vi "Run.vi"(8 "error in (no error)":errorcluster, 11 "Channel in":refnum<class "Channel.lvclass">) -> (0 "error out":errorcluster, 3 "Channel out":refnum<class "Channel.lvclass">)   [LabVIEW 2018, in "Channel.lvclass"]
uses:
  Channel.lvclass
  C:/Users/observer/Desktop/Sparc4GUI/SPARC4_GUI/Device/Device.lvclass
  Channel.lvclass/Channel.ctl
  Interface/Interface.lvclass/Interface.ctl
  Device/Device.lvclass/Device.ctl
  StateMachine/State Machine.lvclass
  Interface/Interface.lvclass
  Device/Device.lvclass
panel:
  out "x = y?":T1
  out "resp ABORT":string
  out "resp STOP":string
  out "resposta do STATUS":string
  out "resp INIT":string
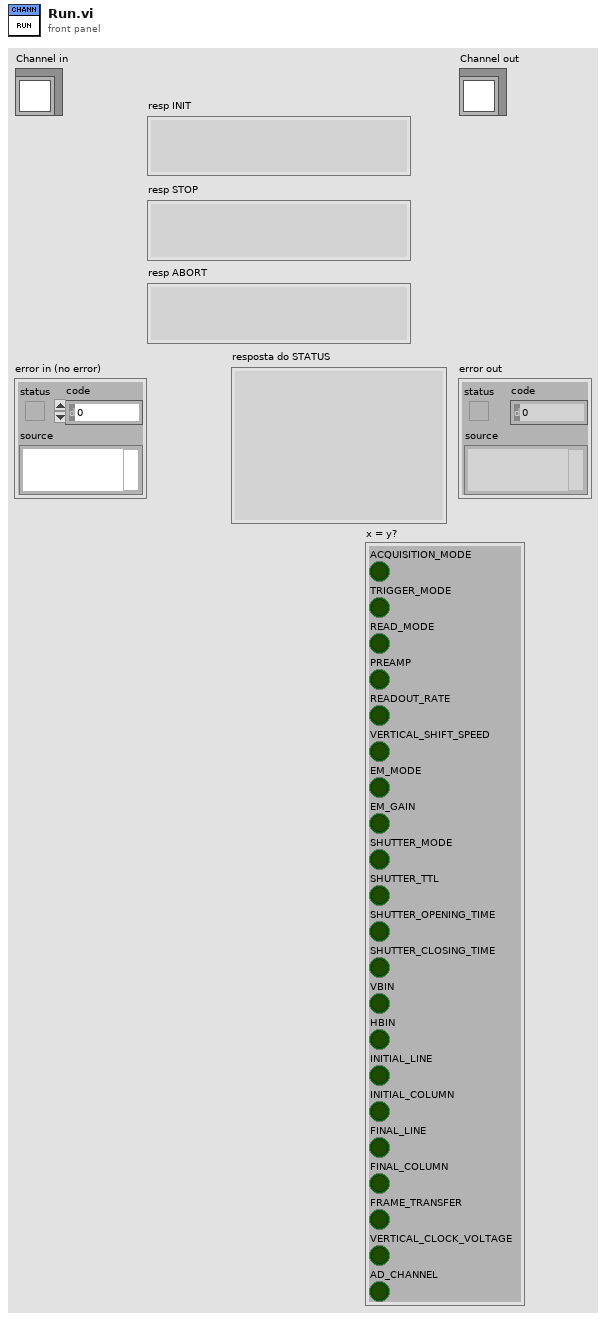
[diagram p1: front panel]
types:
  T1 = cluster{"ACQUISITION_MODE":bool, "TRIGGER_MODE":bool, "READ_MODE":bool, "PREAMP":bool, "READOUT_RATE":bool, "VERTICAL_SHIFT_SPEED":bool, "EM_MODE":bool, "EM_GAIN":bool, "SHUTTER_MODE":bool, "SHUTTER_TTL":bool, "SHUTTER_OPENING_TIME":bool, "SHUTTER_CLOSING_TIME":bool, "VBIN":bool, "HBIN":bool, "INITIAL_LINE":bool, "INITIAL_COLUMN":bool, "FINAL_LINE":bool, "FINAL_COLUMN":bool, "FRAME_TRANSFER":bool, "VERTICAL_CLOCK_VOLTAGE":bool, "AD_CHANNEL":bool}
  T2 = cluster{"ACQUISITION_MODE":u8, "TRIGGER_MODE":u8, "READ_MODE":u8, "PREAMP":u8, "READOUT_RATE":u8, "VERTICAL_SHIFT_SPEED":u8, "EM_MODE":u8, "EM_GAIN":u16, "SHUTTER_MODE":u8, "SHUTTER_TTL":u8, "SHUTTER_OPENING_TIME":u16, "SHUTTER_CLOSING_TIME":u16, "VBIN":u16, "HBIN":u16, "INITIAL_LINE":u16, "INITIAL_COLUMN":u16, "FINAL_LINE":u16, "FINAL_COLUMN":u16, "FRAME_TRANSFER":bool, "VERTICAL_CLOCK_VOLTAGE":u8, "AD_CHANNEL":u32}
  T3 = cluster{"Image Name":string, "Image Path":string, "#FRAMES":u32, "EXPTIME":dbl, "PREAMP":u8, "READOUT_RATE":u8, "VERTICAL_SHIFT_SPEED":u8, "ACQUISITION_MODE":u8, "READ_MODE":u8, "EM_MODE":u8, "EM_GAIN":u16, "SHUTTER_MODE":u8, "SHUTTER_TTL":u8, "SHUTTER_OPENNING_TIME":u16, "SHUTTER_CLOSING_TIME":u16, "VBIN":u16, "HBIN":u16, "INITIAL_LINE":u16, "INITIAL_COLUMN":u16, "FINAL_LINE":u16, "FINAL_COLUMN":u16, "Cooler ON/OFF":u16, "Set temperature":i8, "Exposições realizadas":u16, "Kinetic Serie Length":u32, "Number of Accumulations":u32, "Kinetic Cycle Time":u32, "FRAME_TRANSFER":bool, "VERTICAL_CLOCK_VOLTAGE":u8, "TRIGGER_MODE":u8, "Number of exp":u32, "AD_CHANNEL":u32}
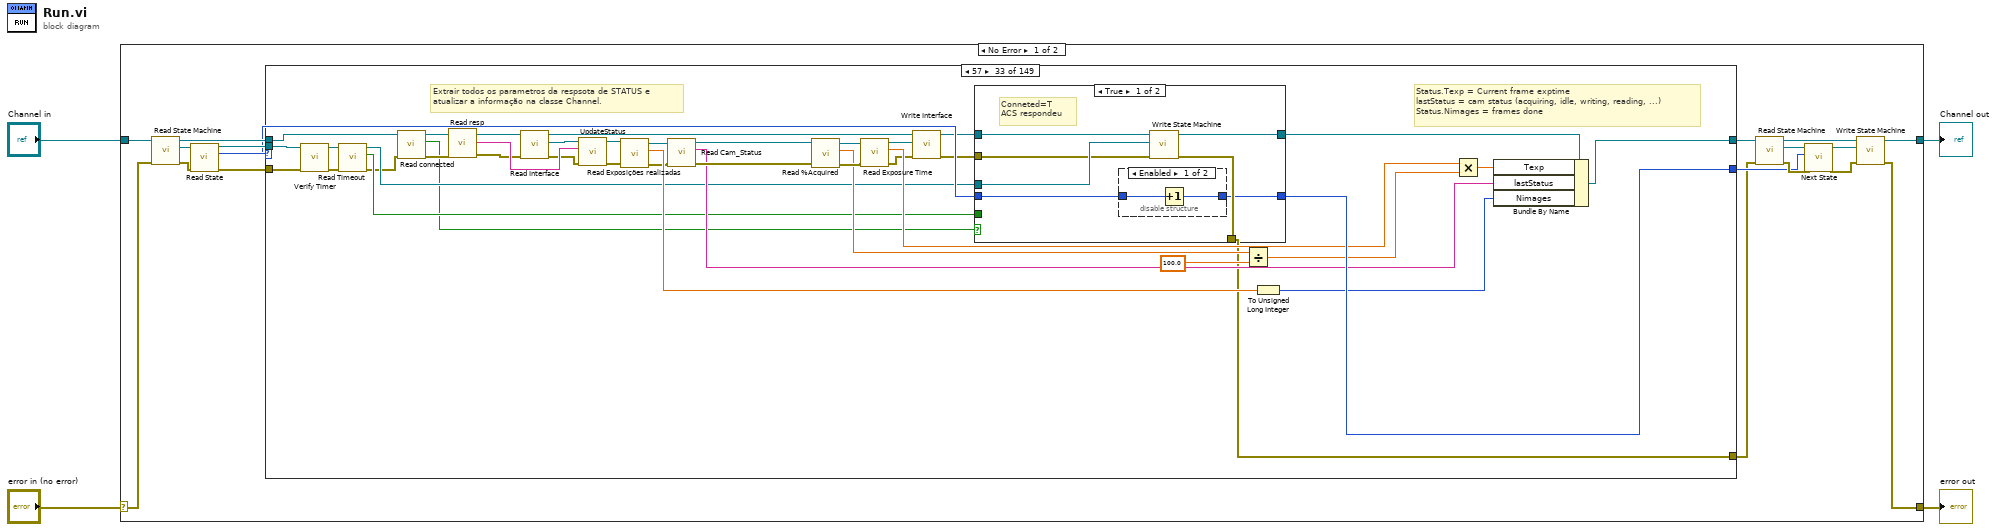
[diagram p0: block diagram]
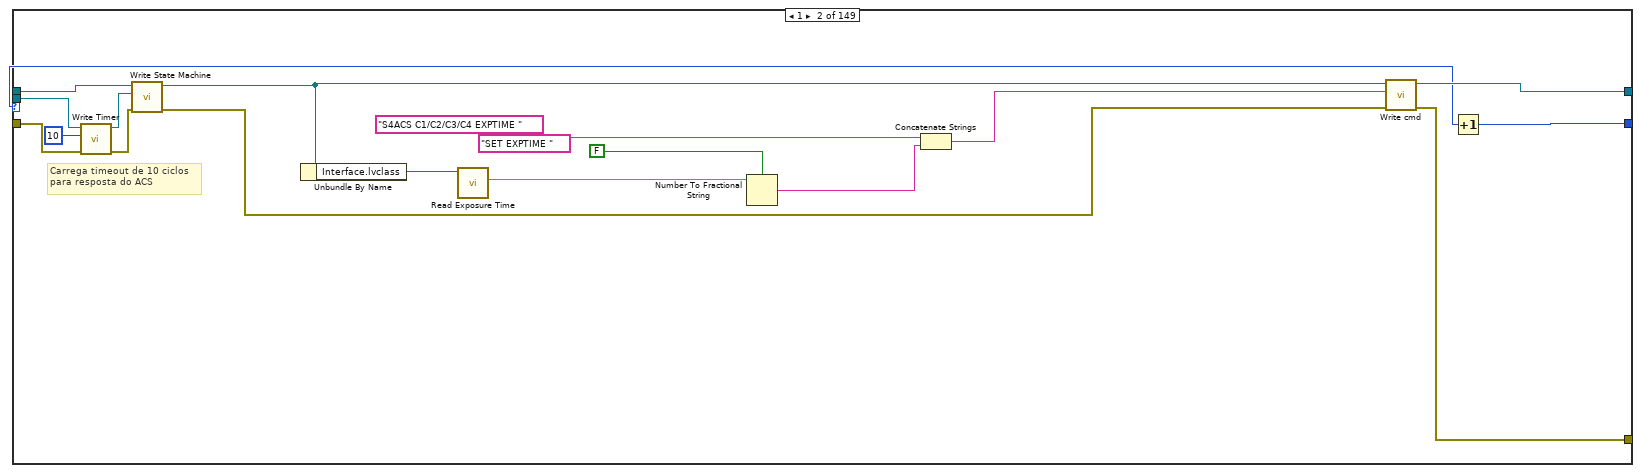
[diagram p3: hidden frame]
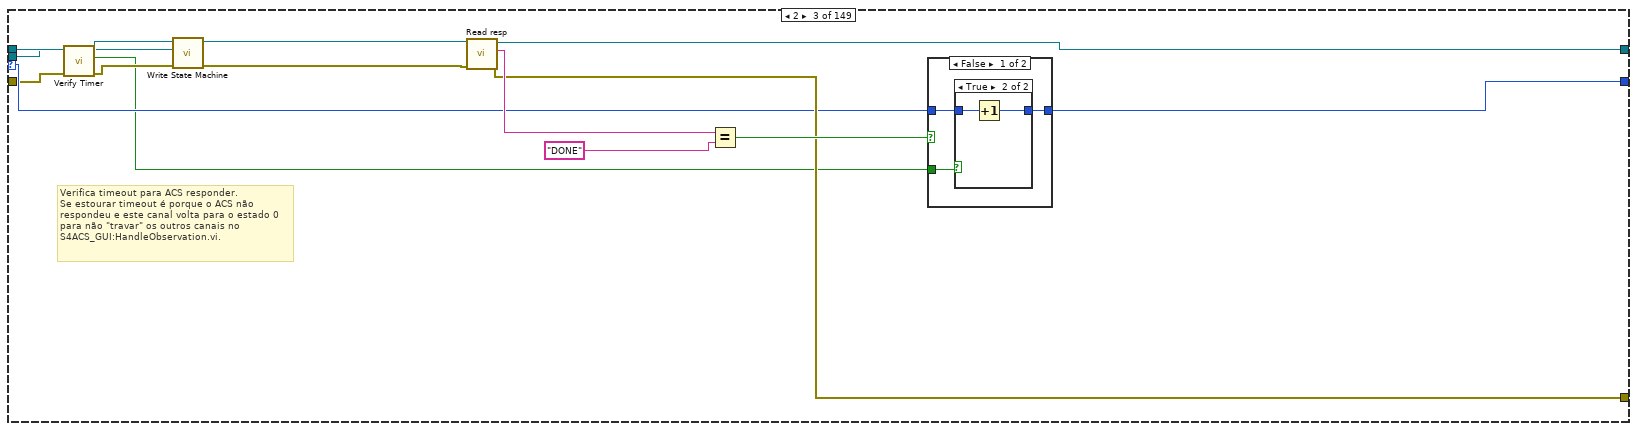
[diagram p4: hidden frame]
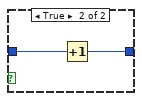
[diagram p6: hidden frame]
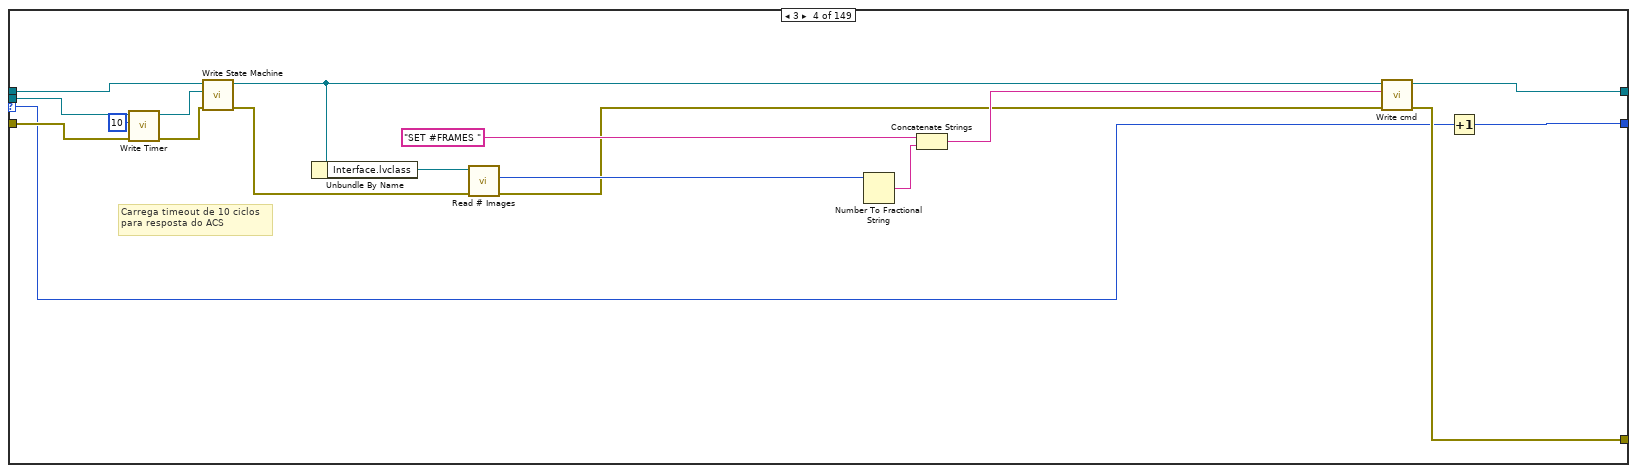
[diagram p7: hidden frame]
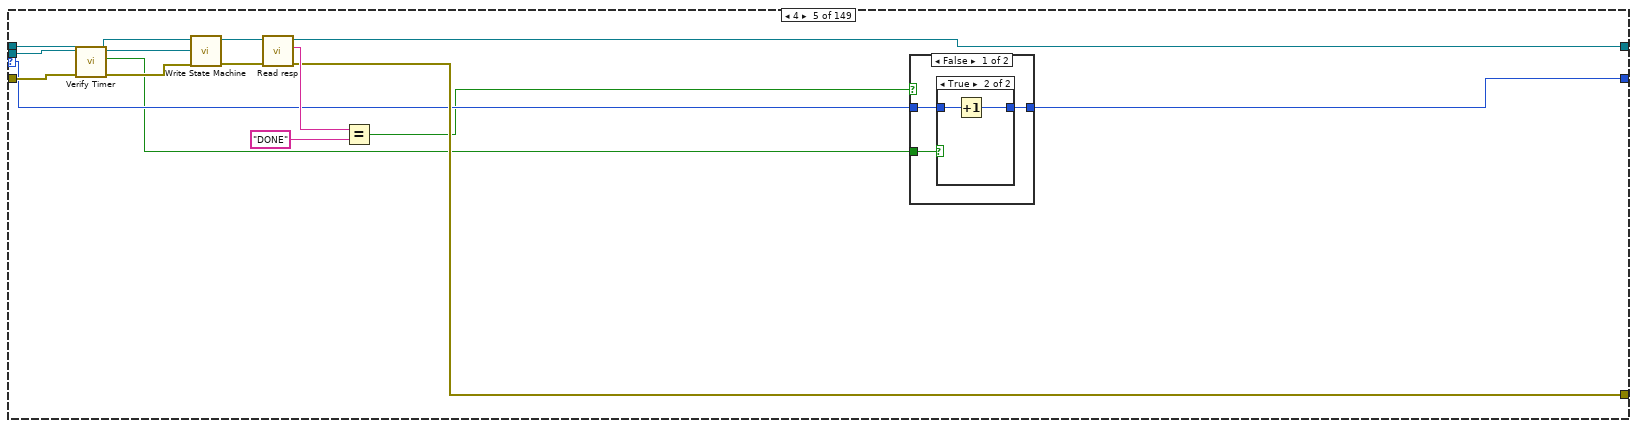
[diagram p8: hidden frame]
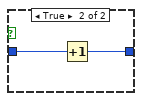
[diagram p10: hidden frame]
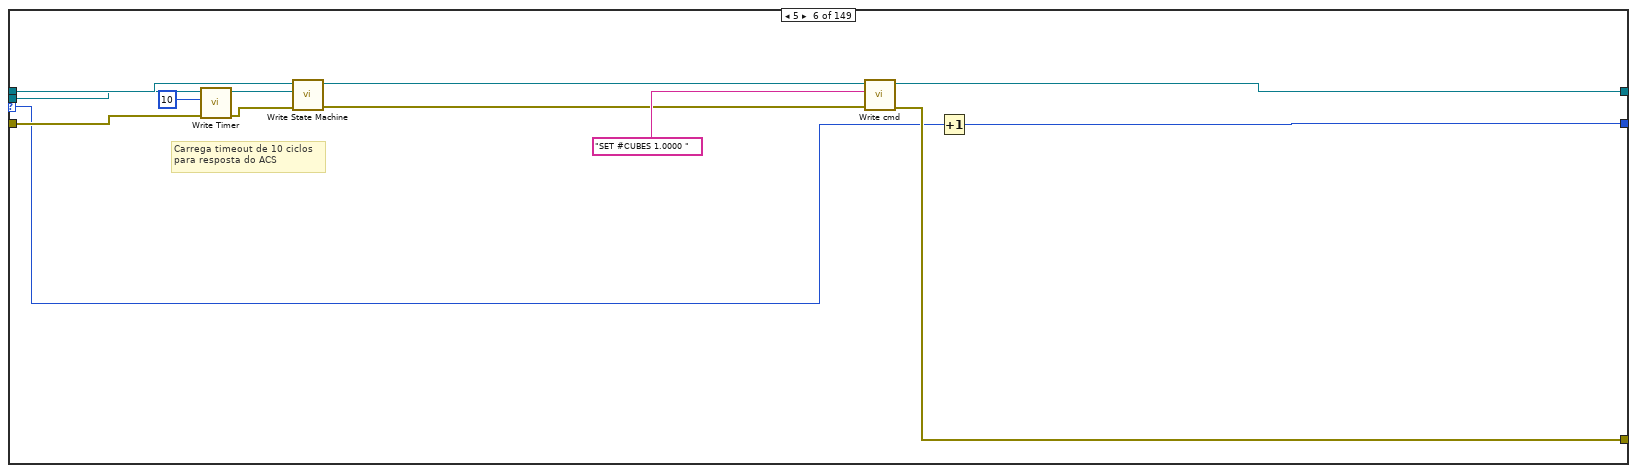
[diagram p11: hidden frame]
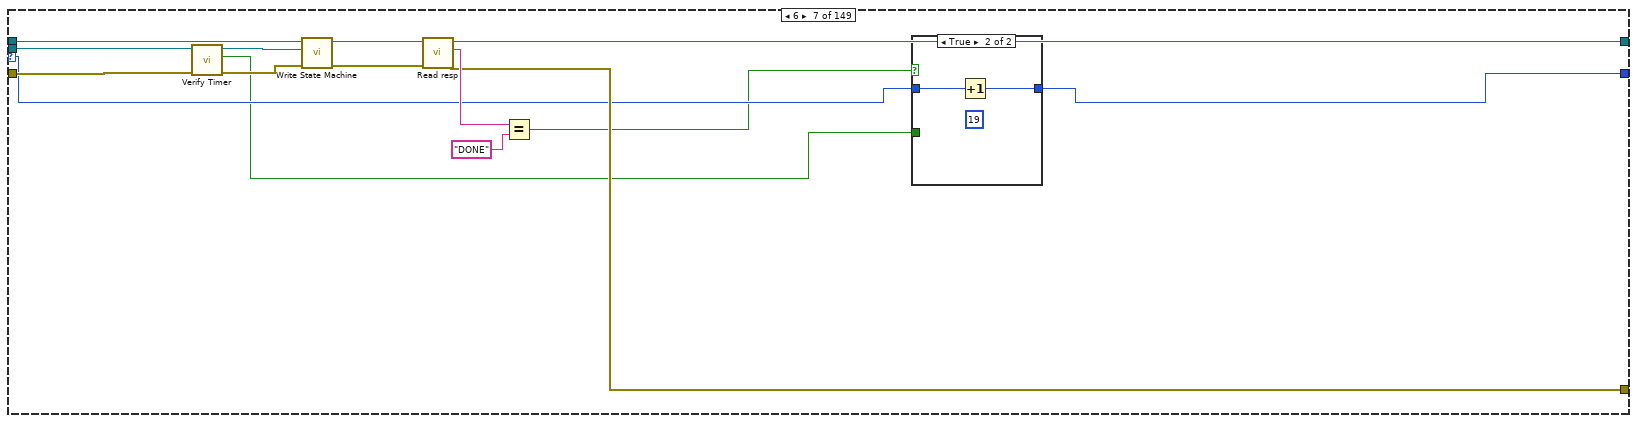
[diagram p12: hidden frame]
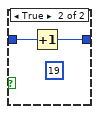
[diagram p14: hidden frame]
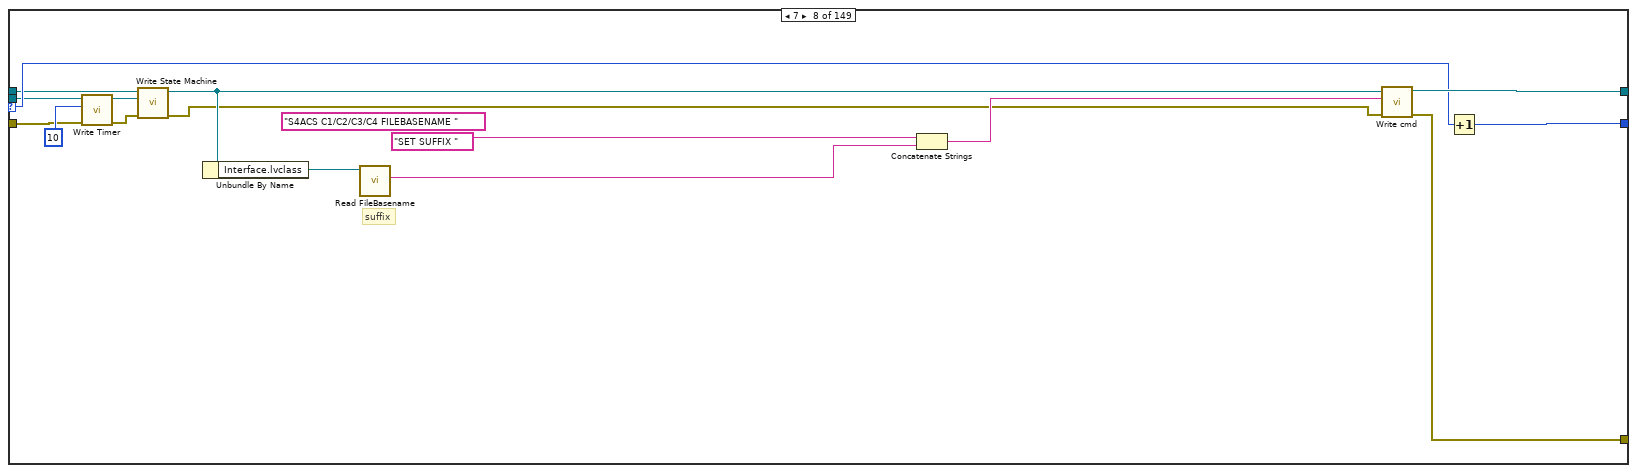
[diagram p15: hidden frame]
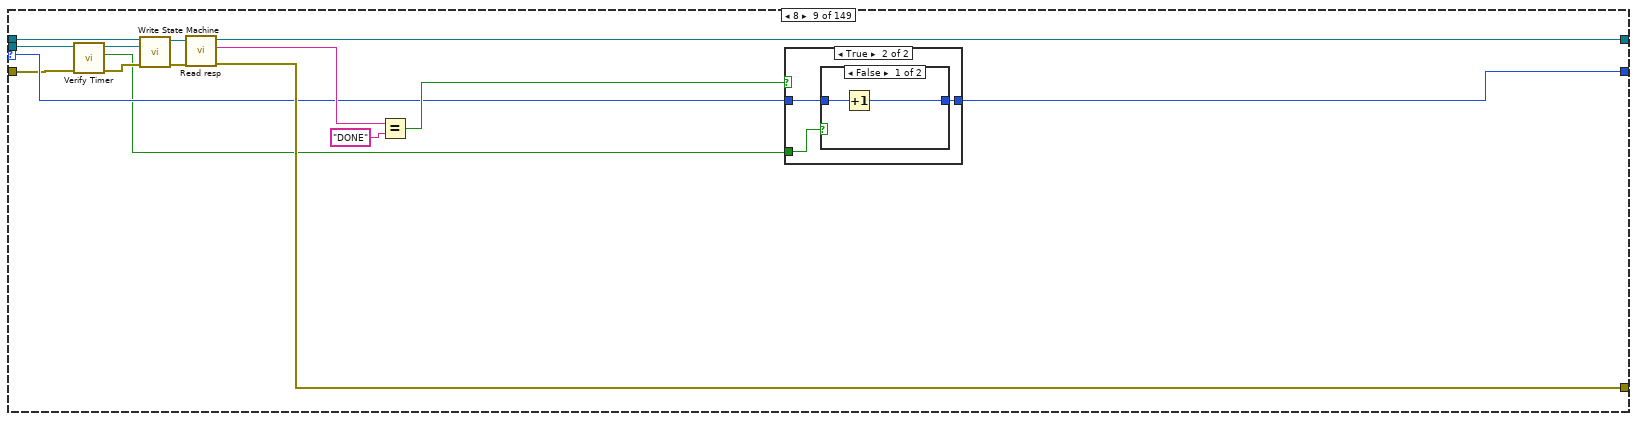
[diagram p16: hidden frame]
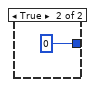
[diagram p18: hidden frame]
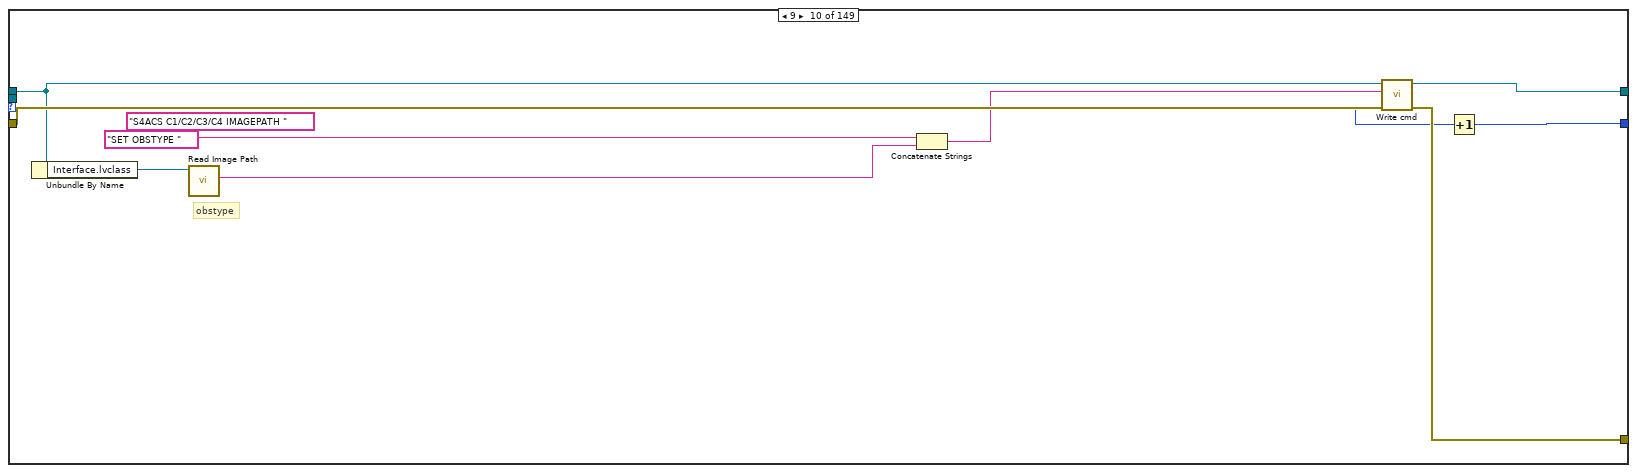
[diagram p19: hidden frame]
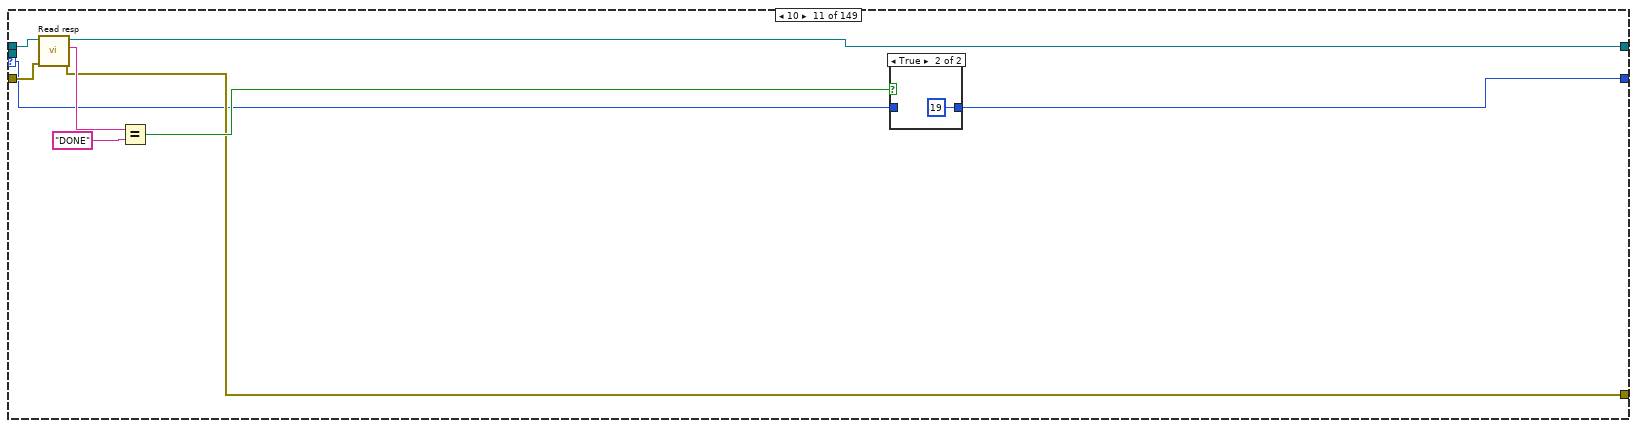
[diagram p20: hidden frame]
diagram:
  n1 = case shown="No Error" "error in (no error)" {
    selector: "error in (no error)" -> [w21 w2224]
    tunnel: [w6 w2224] -> w3
    tunnel: [w11 w2223] -> w1
    tunnel: "Channel in" -> [w22 w2223]
    frame No Error {
      n2 = call-dynamic "Read State Machine.vi"("error in (no error)"=w21, "Device in"=w22) -> ("error out"=w18:errorcluster, "State Machine.lvclass"=w20:refnum<class "State Machine.lvclass">, "Device out"=w16:refnum<class "Channel.lvclass">)  [unwired: 7 in]
      n3 = call-dynamic "Read State.vi"("error in (no error)"=w18, "State Machine in"=w20) -> ("error out"=w17:errorcluster, "State"=w19:i32, "State Machine out"=w5:refnum<class "State Machine.lvclass">)  [unwired: 7 in]
      n4 = case shown="57" w19 {
        selector: w19 -> [w25 w36 w52 w69 w88 w110 w123 w154 w168 w184 w192 w205 w213 w227 w235 w249 w257 w272 w280 w295 w311 w327 w350 w362 _ w420 w431 w445 w484 w502 w541 w598 w647 _ w729 w761 w790 w802 w816 w846 w879 w901 w925 w933 w942 w952 w961 w972 w992 w1012 w1032 w1052 w1072 w1092 w1112 w1132 _ w1152 w1160 w1173 w1186 w1202 w1210 w1223 w1237 w1249 w1257 w1270 w1283 w1295 w1303 w1316 w1329 w1341 w1349 w1362 w1375 w1387 w1395 w1408 w1421 w1433 w1441 w1454 w1467 w1479 w1487 w1500 w1513 w1525 w1533 w1546 w1559 w1575 w1583 w1596 w1609 w1621 w1629 w1642 w1655 w1667 w1675 w1688 w1701 w1713 w1721 w1734 w1747 w1759 w1767 w1780 w1793 w1805 w1813 w1826 w1839 w1851 w1859 w1872 w1885 w1897 w1905 w1918 w1931 w1943 w1951 w1964 w1977 w1989 w1997 w2010 w2023 w2035 w2043 w2056 w2069 w2085 w2093 w2106 w2119 w2131 w2141 w2154 w2167 w2181 w2189 w2202 w2215]
        tunnel: w17 -> [w24 w33 w48 w71 w90 w112 w125 w146 w166 w190 w199 w211 w220 w233 w242 w255 w264 w278 w287 w293 w303 w326 w345 w356 w407 w413 w427 w439 w449 w494 w511 w590 w617 w681 w737 w749 w784 w797 w810 w841 w876 w896 w918 w937 w946 w956 w965 w976 w987 w1007 w1027 w1047 w1067 w1087 w1107 w1127 w1145 w1158 w1167 w1177 w1189 w1208 w1217 w1227 w1240 w1255 w1264 w1274 w1286 w1301 w1310 w1320 w1332 w1347 w1356 w1366 w1378 w1393 w1402 w1412 w1424 w1439 w1448 w1458 w1470 w1485 w1494 w1504 w1516 w1531 w1540 w1550 w1562 w1581 w1590 w1600 w1612 w1627 w1636 w1646 w1658 w1673 w1682 w1692 w1704 w1719 w1728 w1738 w1750 w1765 w1774 w1784 w1796 w1811 w1820 w1830 w1842 w1857 w1866 w1876 w1888 w1903 w1912 w1922 w1934 w1949 w1958 w1968 w1980 w1995 w2004 w2014 w2026 w2041 w2050 w2060 w2072 w2091 w2100 w2110 w2122 w2137 w2148 w2158 w2170 w2187 w2196 w2206 w2218]
        tunnel: [w24 w42 w53 w83 w96 w119 w132 w158 w169 w189 w193 w210 w214 w232 w236 w254 w258 w277 w281 w293 w315 w328 w352 w364 w406 w421 w423 w447 w476 w504 w512 w586 w618 w694 w736 w762 w792 w794 w818 w826 w881 w902 w927 w934 w945 w953 w964 w973 w987 w1007 w1027 w1047 w1067 w1087 w1107 w1127 w1145 w1157 w1161 w1176 w1187 w1207 w1211 w1226 w1238 w1254 w1258 w1273 w1284 w1300 w1304 w1319 w1330 w1346 w1350 w1365 w1376 w1392 w1396 w1411 w1422 w1438 w1442 w1457 w1468 w1484 w1488 w1503 w1514 w1530 w1534 w1549 w1560 w1580 w1584 w1599 w1610 w1626 w1630 w1645 w1656 w1672 w1676 w1691 w1702 w1718 w1722 w1737 w1748 w1764 w1768 w1783 w1794 w1810 w1814 w1829 w1840 w1856 w1860 w1875 w1886 w1902 w1906 w1921 w1932 w1948 w1952 w1967 w1978 w1994 w1998 w2013 w2024 w2040 w2044 w2059 w2070 w2090 w2094 w2109 w2120 w2136 w2142 w2157 w2168 w2186 w2190 w2205 w2216] -> w7
        tunnel: w16 -> [w23 w31 w51 w72 w94 w113 w129 w148 w165 w188 w200 w209 w221 w231 w243 w253 w265 w276 w288 w292 w306 w325 w347 w359 w405 w415 w430 w441 w452 w496 w509 w592 w611 w693 w731 w753 w785 w798 w811 w842 w875 w899 w919 w938 w944 w957 w963 w977 w985 w1005 w1025 w1045 w1065 w1085 w1105 w1125 w1147 w1156 w1168 w1175 w1190 w1206 w1218 w1225 w1241 w1253 w1265 w1272 w1287 w1299 w1311 w1318 w1333 w1345 w1357 w1364 w1379 w1391 w1403 w1410 w1425 w1437 w1449 w1456 w1471 w1483 w1495 w1502 w1517 w1529 w1541 w1548 w1563 w1579 w1591 w1598 w1613 w1625 w1637 w1644 w1659 w1671 w1683 w1690 w1705 w1717 w1729 w1736 w1751 w1763 w1775 w1782 w1797 w1809 w1821 w1828 w1843 w1855 w1867 w1874 w1889 w1901 w1913 w1920 w1935 w1947 w1959 w1966 w1981 w1993 w2005 w2012 w2027 w2039 w2051 w2058 w2073 w2089 w2101 w2108 w2123 w2135 w2149 w2156 w2171 w2185 w2197 w2204 w2219]
        tunnel: [w23 w43 w54 w84 w97 w120 w133 w159 w170 w191 w194 w212 w215 w234 w237 w256 w259 w279 w282 w292 w316 w329 w353 w367 w397 w422 w424 w448 w483 w505 w540 w585 w646 w695 w738 w763 w793 w795 w819 w837 w882 w903 w928 w935 w947 w954 w966 w969 w989 w1009 w1029 w1049 w1069 w1089 w1109 w1129 w1147 w1159 w1162 w1178 w1185 w1209 w1212 w1228 w1236 w1256 w1259 w1275 w1282 w1302 w1305 w1321 w1328 w1348 w1351 w1367 w1374 w1394 w1397 w1413 w1420 w1440 w1443 w1459 w1466 w1486 w1489 w1505 w1512 w1532 w1535 w1551 w1558 w1582 w1585 w1601 w1608 w1628 w1631 w1647 w1654 w1674 w1677 w1693 w1700 w1720 w1723 w1739 w1746 w1766 w1769 w1785 w1792 w1812 w1815 w1831 w1838 w1858 w1861 w1877 w1884 w1904 w1907 w1923 w1930 w1950 w1953 w1969 w1976 w1996 w1999 w2015 w2022 w2042 w2045 w2061 w2068 w2092 w2095 w2111 w2118 w2138 w2143 w2159 w2166 w2188 w2191 w2207 w2214] -> w14
        tunnel: [w25 w37 w55 w78 w85 w118 w124 w155 w171 w185 w195 w206 w216 w228 w238 w250 w260 w273 w283 w296 w312 w330 w351 w363 w399 w410 w432 w446 w485 w503 w542 w599 w648 0 ("State") w728 w764 w791 w803 w817 w847 w880 w904 w926 w936 w943 w955 w962 w974 w984 w1004 w1024 w1044 w1064 w1084 w1104 w1124 u8 0 ("State") w1153 w1163 w1174 w1188 w1203 w1213 w1224 w1239 w1250 w1260 w1271 w1285 w1296 w1306 w1317 w1331 w1342 w1352 w1363 w1377 w1388 w1398 w1409 w1423 w1434 w1444 w1455 w1469 w1480 w1490 w1501 w1515 w1526 w1536 w1547 w1561 w1576 w1586 w1597 w1611 w1622 w1632 w1643 w1657 w1668 w1678 w1689 w1703 w1714 w1724 w1735 w1749 w1760 w1770 w1781 w1795 w1806 w1816 w1827 w1841 w1852 w1862 w1873 w1887 w1898 w1908 w1919 w1933 w1944 w1954 w1965 w1979 w1990 w2000 w2011 w2025 w2036 w2046 w2057 w2071 w2086 w2096 w2107 w2121 w2132 w2144 w2155 w2169 w2182 w2192 w2203 w2217] -> w8
        tunnel: w5 -> [_ w32 w50 w73 w95 w111 w126 w150 w167 _ _ _ _ _ _ _ _ _ _ _ w305 w323 w346 w360 _ w416 w429 w440 w454 w498 w510 w594 w616 w682 w733 w754 w787 w799 w813 w843 w877 w900 w920 _ _ _ _ _ _ _ _ _ _ _ _ _ _ _ _ _ _ _ _ _ _ _ _ _ _ _ _ _ _ _ _ _ _ _ _ _ _ _ _ _ _ _ _ _ _ _ _ _ _ _ _ _ _ _ _ _ _ _ _ _ _ _ _ _ _ _ _ _ _ _ _ _ _ _ _ _ _ _ _ _ _ _ _ _ _ _ _ _ _ _ _ _ _ _ _ _ _ _ _ _ _ _ _ _ _]
        frame 0, Default {
        }
        frame 1 {
          (unwired) "S4ACS C1/C2/C3/C4 EXPTIME " ("cmd")
          # "Carrega timeout de 10 ciclos\npara resposta do ACS"
          n5 = call-dynamic "Write Timer.vi"("error in (no error)"=w33, "Timer"=u32 10, "State Machine in"=w32) -> ("error out"=w27:errorcluster, "State Machine out"=w30:refnum<class "State Machine.lvclass">)  [unwired: 7 in]
          n6 = call-dynamic "Write State Machine.vi"("error in (no error)"=w27, "State Machine.lvclass"=w30, "Device in"=w31) -> ("error out"=w26:errorcluster, "Device out"=w29:refnum<class "Channel.lvclass">)  [unwired: 7 in]
          n7 = Unbundle By Name(w29) -> ("Interface.lvclass"=w41:refnum<class "Interface.lvclass">)
          n8 = call "Read Exposure Time.vi"("Interface in"=w41) -> ("Exposure Time"=w40:dbl)  [unwired: 8 in, 2 out]
          n9 = Number To Fractional String(use system decimal point (T)=FALSE, number=w40) -> (F-format string=w39:string)  [unwired: 2 in]
          n10 = Concatenate Strings("SET EXPTIME " ("cmd"), w39) -> (w38:string)
          n11 = call-dynamic "Write cmd.vi"("error in (no error)"=w26, "cmd"=w38, "Device in"=w29) -> ("error out"=w42:errorcluster, "Device out"=w43:refnum<class "Channel.lvclass">)  [unwired: 7 in]
          n12 = Increment(x=w36) -> (x+1=w37:i32)
        }
        frame 2 {
          # "Verifica timeout para ACS responder.\nSe estourar timeout é porque o ACS não \nrespondeu e este canal volta para o estado 0\npara não \"travar\" os outros canais no \nS4ACS_GUI:HandleObservation.vi."
          n13 = call "Verify Timer.vi"("error in (no error)"=w48, "State Machine in"=w50) -> ("error out"=w47:errorcluster, "timeout"=w44:bool, "State Machine out"=w49:refnum<class "State Machine.lvclass">)  [unwired: 7 in]
          n14 = call-dynamic "Write State Machine.vi"("error in (no error)"=w47, "State Machine.lvclass"=w49, "Device in"=w51) -> ("error out"=w46:errorcluster, "Device out"=w45:refnum<class "Channel.lvclass">)  [unwired: 7 in]
          n15 = call-dynamic "Read resp.vi"("error in (no error)"=w46, "Device in"=w45) -> ("error out"=w53:errorcluster, "resp"=w58:string, "Device out"=w54:refnum<class "Channel.lvclass">)  [unwired: 7 in]
          n16 = Equal?(x=w58, y="DONE") -> (x = y?=w56:bool)
          n17 = case shown="False" w56 {
            tunnel: [w60 w65] -> w55
            tunnel: w52 -> [w61 w66]
            tunnel: w44 -> [w59 _]
            frame False {
              n18 = case shown="True" w59 {
                tunnel: [w62 w63] -> w60
                tunnel: w61 -> [w62 w64]
                frame False {
                }
                frame True {
                  n19 = Increment(x=w64) -> (x+1=w63:i32)
                }
              }
            }
            frame True {
              n20 = Increment(x=w66) -> (x+1=w65:i32)
            }
          }
        }
        frame 3 {
          # "Carrega timeout de 10 ciclos\npara resposta do ACS"
          n21 = call-dynamic "Write Timer.vi"("error in (no error)"=w71, "Timer"=u32 10, "State Machine in"=w73) -> ("error out"=w74:errorcluster, "State Machine out"=w76:refnum<class "State Machine.lvclass">)  [unwired: 7 in]
          n22 = call-dynamic "Write State Machine.vi"("error in (no error)"=w74, "State Machine.lvclass"=w76, "Device in"=w72) -> ("error out"=w68:errorcluster, "Device out"=w70:refnum<class "Channel.lvclass">)  [unwired: 7 in]
          n23 = Unbundle By Name(w70) -> ("Interface.lvclass"=w82:refnum<class "Interface.lvclass">)
          n24 = call-dynamic "Read # Images.vi"("error in (no error)"=w68, "Interface in"=w82) -> ("error out"=w67:errorcluster, "# Images"=w81:u32)  [unwired: 7 in, 1 out]
          n25 = Number To Fractional String(number=w81) -> (F-format string=w80:string)  [unwired: 3 in]
          n26 = Concatenate Strings("SET #FRAMES " ("cmd"), w80) -> (w79:string)
          n27 = call-dynamic "Write cmd.vi"("error in (no error)"=w67, "cmd"=w79, "Device in"=w70) -> ("error out"=w83:errorcluster, "Device out"=w84:refnum<class "Channel.lvclass">)  [unwired: 7 in]
          n28 = Increment(x=w69) -> (x+1=w78:i32)
        }
        frame 4 {
          n29 = call "Verify Timer.vi"("error in (no error)"=w90, "State Machine in"=w95) -> ("error out"=w89:errorcluster, "timeout"=w86:bool, "State Machine out"=w91:refnum<class "State Machine.lvclass">)  [unwired: 7 in]
          n30 = call-dynamic "Write State Machine.vi"("error in (no error)"=w89, "State Machine.lvclass"=w91, "Device in"=w94) -> ("error out"=w92:errorcluster, "Device out"=w93:refnum<class "Channel.lvclass">)  [unwired: 7 in]
          n31 = call-dynamic "Read resp.vi"("error in (no error)"=w92, "Device in"=w93) -> ("error out"=w96:errorcluster, "resp"=w99:string, "Device out"=w97:refnum<class "Channel.lvclass">)  [unwired: 7 in]
          n32 = Equal?(x=w99, y="DONE") -> (x = y?=w87:bool)
          n33 = case shown="False" w87 {
            tunnel: [w101 w106] -> w85
            tunnel: w88 -> [w102 w107]
            tunnel: w86 -> [w100 _]
            frame False {
              n34 = case shown="True" w100 {
                tunnel: [w103 w104] -> w101
                tunnel: w102 -> [w103 w105]
                frame False {
                }
                frame True {
                  n35 = Increment(x=w105) -> (x+1=w104:i32)
                }
              }
            }
            frame True {
              n36 = Increment(x=w107) -> (x+1=w106:i32)
            }
          }
        }
        frame 5 {
          # "Carrega timeout de 10 ciclos\npara resposta do ACS"
          n37 = call-dynamic "Write Timer.vi"("error in (no error)"=w112, "Timer"=u32 10, "State Machine in"=w111) -> ("error out"=w114:errorcluster, "State Machine out"=w116:refnum<class "State Machine.lvclass">)  [unwired: 7 in]
          n38 = call-dynamic "Write State Machine.vi"("error in (no error)"=w114, "State Machine.lvclass"=w116, "Device in"=w113) -> ("error out"=w109:errorcluster, "Device out"=w108:refnum<class "Channel.lvclass">)  [unwired: 7 in]
          n39 = call-dynamic "Write cmd.vi"("error in (no error)"=w109, "cmd"="SET #CUBES 1.0000 ", "Device in"=w108) -> ("error out"=w119:errorcluster, "Device out"=w120:refnum<class "Channel.lvclass">)  [unwired: 7 in]
          n40 = Increment(x=w110) -> (x+1=w118:i32)
        }
        frame 6 {
          n41 = call "Verify Timer.vi"("error in (no error)"=w125, "State Machine in"=w126) -> ("error out"=w130:errorcluster, "timeout"=w121:bool, "State Machine out"=w131:refnum<class "State Machine.lvclass">)  [unwired: 7 in]
          n42 = call-dynamic "Write State Machine.vi"("error in (no error)"=w130, "State Machine.lvclass"=w131, "Device in"=w129) -> ("error out"=w127:errorcluster, "Device out"=w128:refnum<class "Channel.lvclass">)  [unwired: 7 in]
          n43 = call-dynamic "Read resp.vi"("error in (no error)"=w127, "Device in"=w128) -> ("error out"=w132:errorcluster, "resp"=w135:string, "Device out"=w133:refnum<class "Channel.lvclass">)  [unwired: 7 in]
          n44 = Equal?(x=w135, y="DONE") -> (x = y?=w122:bool)
          n45 = case shown="True" w122 {
            tunnel: [w137 w142] -> w124
            tunnel: w123 -> [w138 w143]
            tunnel: w121 -> [w136 _]
            frame False {
              n46 = case shown="False" w136 {
                tunnel: [w139 w140] -> w137
                tunnel: w138 -> [w139 w141]
                frame False {
                }
                frame True {
                  (unwired) 19 ("State")
                  n47 = Increment(x=w141) -> (x+1=w140:i32)
                }
              }
            }
            frame True {
              (unwired) 19
              n48 = Increment(x=w143) -> (x+1=w142:i32)
            }
          }
        }
        frame 7 {
          (unwired) "S4ACS C1/C2/C3/C4 FILEBASENAME " ("cmd")
          # "suffix"
          n49 = call-dynamic "Write Timer.vi"("error in (no error)"=w146, "Timer"=u32 10, "State Machine in"=w150) -> ("error out"=w151:errorcluster, "State Machine out"=w144:refnum<class "State Machine.lvclass">)  [unwired: 7 in]
          n50 = call-dynamic "Write State Machine.vi"("error in (no error)"=w151, "State Machine.lvclass"=w144, "Device in"=w148) -> ("error out"=w145:errorcluster, "Device out"=w147:refnum<class "Channel.lvclass">)  [unwired: 7 in]
          n51 = Unbundle By Name(w147) -> ("Interface.lvclass"=w157:refnum<class "Interface.lvclass">)
          n52 = call-dynamic "Read FileBasename.vi"("Interface in"=w157) -> ("FileBasename"=w152:string)  [unwired: 8 in, 2 out]
          n53 = Concatenate Strings("SET SUFFIX " ("cmd"), w152) -> (w156:string)
          n54 = call-dynamic "Write cmd.vi"("error in (no error)"=w145, "cmd"=w156, "Device in"=w147) -> ("error out"=w158:errorcluster, "Device out"=w159:refnum<class "Channel.lvclass">)  [unwired: 7 in]
          n55 = Increment(x=w154) -> (x+1=w155:i32)
        }
        frame 8 {
          n56 = call "Verify Timer.vi"("error in (no error)"=w166, "State Machine in"=w167) -> ("error out"=w163:errorcluster, "timeout"=w160:bool, "State Machine out"=w164:refnum<class "State Machine.lvclass">)  [unwired: 7 in]
          n57 = call-dynamic "Write State Machine.vi"("error in (no error)"=w163, "State Machine.lvclass"=w164, "Device in"=w165) -> ("error out"=w162:errorcluster, "Device out"=w161:refnum<class "Channel.lvclass">)  [unwired: 7 in]
          n58 = call-dynamic "Read resp.vi"("error in (no error)"=w162, "Device in"=w161) -> ("error out"=w169:errorcluster, "resp"=w174:string, "Device out"=w170:refnum<class "Channel.lvclass">)  [unwired: 7 in]
          n59 = Equal?(x=w174, y="DONE") -> (x = y?=w172:bool)
          n60 = case shown="True" w172 {
            tunnel: [w175 w177] -> w171
            tunnel: w168 -> [w175 w178]
            tunnel: w160 -> [_ w176]
            frame False {
            }
            frame True {
              n61 = case shown="False" w176 {
                tunnel: w178 -> [w180 _]
                tunnel: [w179 0] -> w177
                frame False {
                  n62 = Increment(x=w180) -> (x+1=w179:i32)
                }
                frame True {
                }
              }
            }
          }
        }
        frame 9 {
          (unwired) "S4ACS C1/C2/C3/C4 IMAGEPATH " ("cmd")
          # "obstype"
          n63 = Unbundle By Name(w188) -> ("Interface.lvclass"=w187:refnum<class "Interface.lvclass">)
          n64 = call-dynamic "Read Image Path.vi"("Interface in"=w187) -> ("Image Path"=w182:string)  [unwired: 8 in, 2 out]
          n65 = Concatenate Strings("SET OBSTYPE " ("cmd"), w182) -> (w186:string)
          n66 = call-dynamic "Write cmd.vi"("error in (no error)"=w190, "cmd"=w186, "Device in"=w188) -> ("error out"=w189:errorcluster, "Device out"=w191:refnum<class "Channel.lvclass">)  [unwired: 7 in]
          n67 = Increment(x=w184) -> (x+1=w185:i32)
        }
        frame 10 {
          n68 = call-dynamic "Read resp.vi"("error in (no error)"=w199, "Device in"=w200) -> ("error out"=w193:errorcluster, "resp"=w198:string, "Device out"=w194:refnum<class "Channel.lvclass">)  [unwired: 7 in]
          n69 = Equal?(x=w198, y="DONE") -> (x = y?=w196:bool)
          n70 = case shown="True" w196 {
            tunnel: [w201 19 ("State")] -> w195
            tunnel: w192 -> [w201 _]
            frame False {
            }
            frame True {
            }
          }
        }
        frame 11 {
          (unwired) "S4ACS C1/C2/C3/C4 OBSTITLE " ("cmd")
          n71 = Unbundle By Name(w209) -> ("Interface.lvclass"=w208:refnum<class "Interface.lvclass">)
          n72 = call-dynamic "Read ObsTitle.vi"("Interface in"=w208) -> ("ObsTitle"=w203:string)  [unwired: 8 in, 2 out]
          n73 = Concatenate Strings("SET OBSERVATION_TITLE " ("cmd"), w203) -> (w207:string)
          n74 = call-dynamic "Write cmd.vi"("error in (no error)"=w211, "cmd"=w207, "Device in"=w209) -> ("error out"=w210:errorcluster, "Device out"=w212:refnum<class "Channel.lvclass">)  [unwired: 7 in]
          n75 = Increment(x=w205) -> (x+1=w206:i32)
        }
        frame 12 {
          n76 = call-dynamic "Read resp.vi"("error in (no error)"=w220, "Device in"=w221) -> ("error out"=w214:errorcluster, "resp"=w219:string, "Device out"=w215:refnum<class "Channel.lvclass">)  [unwired: 7 in]
          n77 = Equal?(x=w219, y="DONE") -> (x = y?=w217:bool)
          n78 = case shown="True" w217 {
            tunnel: [w222 w223] -> w216
            tunnel: w213 -> [w222 w224]
            frame False {
            }
            frame True {
              n79 = Increment(x=w224) -> (x+1=w223:i32)
            }
          }
        }
        frame 13 {
          (unwired) "S4ACS C1/C2/C3/C4 COMMENTS " ("cmd")
          n80 = Unbundle By Name(w231) -> ("Interface.lvclass"=w230:refnum<class "Interface.lvclass">)
          n81 = call-dynamic "Read Comments.vi"("Interface in"=w230) -> ("Comments"=w225:string)  [unwired: 8 in, 2 out]
          n82 = Concatenate Strings("SET COMMENT " ("cmd"), w225) -> (w229:string)
          n83 = call-dynamic "Write cmd.vi"("error in (no error)"=w233, "cmd"=w229, "Device in"=w231) -> ("error out"=w232:errorcluster, "Device out"=w234:refnum<class "Channel.lvclass">)  [unwired: 7 in]
          n84 = Increment(x=w227) -> (x+1=w228:i32)
        }
        frame 14 {
          n85 = call-dynamic "Read resp.vi"("error in (no error)"=w242, "Device in"=w243) -> ("error out"=w236:errorcluster, "resp"=w241:string, "Device out"=w237:refnum<class "Channel.lvclass">)  [unwired: 7 in]
          n86 = Equal?(x=w241, y="DONE") -> (x = y?=w239:bool)
          n87 = case shown="True" w239 {
            tunnel: [w244 w245] -> w238
            tunnel: w235 -> [w244 w246]
            frame False {
            }
            frame True {
              n88 = Increment(x=w246) -> (x+1=w245:i32)
            }
          }
        }
        frame 15 {
          (unwired) "S4ACS C1/C2/C3/C4 DS9 " ("cmd")
          n89 = Unbundle By Name(w253) -> ("Interface.lvclass"=w252:refnum<class "Interface.lvclass">)
          n90 = call-dynamic "Read DS9.vi"("Interface in"=w252) -> ("DS9"=w247:string)  [unwired: 8 in, 2 out]
          n91 = Concatenate Strings("SET DS9 " ("cmd"), w247) -> (w251:string)
          n92 = call-dynamic "Write cmd.vi"("error in (no error)"=w255, "cmd"=w251, "Device in"=w253) -> ("error out"=w254:errorcluster, "Device out"=w256:refnum<class "Channel.lvclass">)  [unwired: 7 in]
          n93 = Increment(x=w249) -> (x+1=w250:i32)
        }
        frame 16 {
          n94 = call-dynamic "Read resp.vi"("error in (no error)"=w264, "Device in"=w265) -> ("error out"=w258:errorcluster, "resp"=w263:string, "Device out"=w259:refnum<class "Channel.lvclass">)  [unwired: 7 in]
          n95 = Equal?(x=w263, y="DONE") -> (x = y?=w261:bool)
          n96 = case shown="True" w261 {
            tunnel: [w266 w267] -> w260
            tunnel: w257 -> [w266 w268]
            frame False {
            }
            frame True {
              n97 = Increment(x=w268) -> (x+1=w267:i32)
            }
          }
        }
        frame 17 {
          (unwired) "S4ACS C1/C2/C3/C4 DS9 " ("cmd")
          n98 = Unbundle By Name(w276) -> ("Interface.lvclass"=w275:refnum<class "Interface.lvclass">)
          n99 = call "Read Kinetic Series Length.vi"("Interface in"=w275) -> ("Kinetic Series Length"=w270:u32)  [unwired: 8 in, 2 out]
          n100 = Number To Decimal String(number=w270) -> (decimal integer string=w269:string)  [unwired: 1 in]
          n101 = Concatenate Strings("SET KSERLEN " ("cmd"), w269) -> (w274:string)
          n102 = call-dynamic "Write cmd.vi"("error in (no error)"=w278, "cmd"=w274, "Device in"=w276) -> ("error out"=w277:errorcluster, "Device out"=w279:refnum<class "Channel.lvclass">)  [unwired: 7 in]
          n103 = Increment(x=w272) -> (x+1=w273:i32)
        }
        frame 18 {
          n104 = call-dynamic "Read resp.vi"("error in (no error)"=w287, "Device in"=w288) -> ("error out"=w281:errorcluster, "resp"=w286:string, "Device out"=w282:refnum<class "Channel.lvclass">)  [unwired: 7 in]
          n105 = Equal?(x=w286, y="DONE") -> (x = y?=w284:bool)
          n106 = case shown="True" w284 {
            tunnel: [w289 w290] -> w283
            tunnel: w280 -> [w289 w291]
            frame False {
            }
            frame True {
              n107 = Increment(x=w291) -> (x+1=w290:i32)
            }
          }
        }
        frame 19 {
          n108 = Unbundle By Name(w292) -> ("expose"=w294:bool)
          n109 = case shown="False" w294 {
            tunnel: [u8 0 ("State") u8 50 ("State")] -> w296
            tunnel: w295 -> [_ _]
            frame False {
            }
            frame True {
            }
          }
        }
        frame 30 {
          n110 = call-dynamic "Write Timer.vi"("error in (no error)"=w303, "Timer"=u32 50, "State Machine in"=w305) -> ("error out"=w302:errorcluster, "State Machine out"=w304:refnum<class "State Machine.lvclass">)  [unwired: 7 in]
          n111 = call-dynamic "Write State Machine.vi"("error in (no error)"=w302, "State Machine.lvclass"=w304, "Device in"=w306) -> ("error out"=w300:errorcluster, "Device out"=w301:refnum<class "Channel.lvclass">)  [unwired: 7 in]
          n112 = Unbundle By Name(w301) -> ("Interface.lvclass"=w314:refnum<class "Interface.lvclass">)
          n113 = call-dynamic "Read Cooler ON_OFF.vi"("error in (no error)"=w300, "Interface in"=w314) -> ("error out"=w299:errorcluster, "Cooler ON/OFF"=w309:i16)  [unwired: 7 in, 1 out]
          n114 = case shown="1, Default" w309 {
            tunnel: ["1" "0"] -> w308
            frame 0 {
              (unwired) "ON"
              # "Se COOLER desligado, manda ligar."
            }
            frame 1, Default {
              (unwired) "OFF"
              # "Se COOLER ligado, manda desligar."
            }
          }
          n115 = Concatenate Strings("SET COOLER_POWER_STATUS " ("cmd"), w308) -> (w313:string)
          n116 = call-dynamic "Write cmd.vi"("error in (no error)"=w299, "cmd"=w313, "Device in"=w301) -> ("error out"=w315:errorcluster, "Device out"=w316:refnum<class "Channel.lvclass">)  [unwired: 7 in]
          n117 = Increment(x=w311) -> (x+1=w312:i32)
        }
        frame 31 {
          n118 = call "Verify Timer.vi"("error in (no error)"=w326, "State Machine in"=w323) -> ("error out"=w321:errorcluster, "timeout"=w319:bool, "State Machine out"=w322:refnum<class "State Machine.lvclass">)  [unwired: 7 in]
          n119 = call-dynamic "Write State Machine.vi"("error in (no error)"=w321, "State Machine.lvclass"=w322, "Device in"=w325) -> ("error out"=w320:errorcluster, "Device out"=w324:refnum<class "Channel.lvclass">)  [unwired: 7 in]
          n120 = call-dynamic "Read resp.vi"("error in (no error)"=w320, "Device in"=w324) -> ("error out"=w328:errorcluster, "resp"=w333:string, "Device out"=w329:refnum<class "Channel.lvclass">)  [unwired: 7 in]
          n121 = Equal?(x=w333, y="DONE") -> (x = y?=w331:bool)
          n122 = case shown="False" w319 {
            tunnel: w331 -> [w336 _]
            tunnel: [w335 0 ("State")] -> w330
            tunnel: w327 -> [w334 _]
            frame False {
              n123 = case shown="True" w336 {
                tunnel: [w337 w338] -> w335
                tunnel: w334 -> [w337 w339]
                frame False {
                }
                frame True {
                  n124 = Increment(x=w339) -> (x+1=w338:i32)
                }
              }
            }
            frame True {
            }
          }
        }
        frame 32 {
          n125 = call-dynamic "Write Timer.vi"("error in (no error)"=w345, "Timer"=u32 50, "State Machine in"=w346) -> ("error out"=w348:errorcluster, "State Machine out"=w343:refnum<class "State Machine.lvclass">)  [unwired: 7 in]
          n126 = call-dynamic "Write State Machine.vi"("error in (no error)"=w348, "State Machine.lvclass"=w343, "Device in"=w347) -> ("error out"=w341:errorcluster, "Device out"=w342:refnum<class "Channel.lvclass">)  [unwired: 7 in]
          n127 = call-dynamic "Write cmd.vi"("error in (no error)"=w341, "cmd"="GET COOLER_POWER_STATUS ", "Device in"=w342) -> ("error out"=w352:errorcluster, "Device out"=w353:refnum<class "Channel.lvclass">)  [unwired: 7 in]
          n128 = Increment(x=w350) -> (x+1=w351:i32)
        }
        frame 33 {
          n129 = call "Verify Timer.vi"("error in (no error)"=w356, "State Machine in"=w360) -> ("error out"=w355:errorcluster, "timeout"=w354:bool, "State Machine out"=w357:refnum<class "State Machine.lvclass">)  [unwired: 7 in]
          n130 = call-dynamic "Write State Machine.vi"("error in (no error)"=w355, "State Machine.lvclass"=w357, "Device in"=w359) -> ("Device out"=w358:refnum<class "Channel.lvclass">)  [unwired: 7 in, 1 out]
          n131 = call-dynamic "Read resp.vi"("Device in"=w358) -> ("error out"=w365:errorcluster, "resp"=w361:string, "Device out"=w366:refnum<class "Channel.lvclass">)  [unwired: 8 in]
          n132 = case shown="False" w354 {
            tunnel: [w374 w393] -> w367
            tunnel: w366 -> [w373 w393]
            tunnel: w365 -> [w372 w392]
            tunnel: [w371 w392] -> w364
            tunnel: [w370 0 ("State")] -> w363
            tunnel: w362 -> [w369 _]
            tunnel: w361 -> [w368 _]
            frame False {
              n133 = case shown="Default" w368 {
                selector: w368 -> [_ w386]
                tunnel: [w377 w382] -> w374
                tunnel: w373 -> [w377 w390]
                tunnel: w372 -> [w376 w388]
                tunnel: [w376 w380] -> w371
                tunnel: [w375 0 ("State")] -> w370
                tunnel: w369 -> [w375 _]
                frame Default {
                }
                frame "0", "1" {
                  n134 = Decimal String To Number(string=w386) -> (number=w385:i32)  [unwired: 2 in, 1 out]
                  n135 = Unbundle By Name(w390) -> ("Interface.lvclass"=w389:refnum<class "Interface.lvclass">)
                  n136 = To Word Integer(number=w385) -> (16bit integer=w384:i16)
                  n137 = call-dynamic "Write Cooler ON_OFF.vi"("error in (no error)"=w388, "Cooler ON/OFF"=w384, "Interface in"=w389) -> ("error out"=w381:errorcluster, "Interface out"=w379:refnum<class "Interface.lvclass">)  [unwired: 7 in]
                  n138 = Bundle By Name(cluster=w390, "Interface.lvclass"=w379) -> (w383:refnum<class "Channel.lvclass">)
                  n139 = call-dynamic "Save Temp.vi"("error in (no error)"=w381, "temp file"="lasttemp.cfg", "Channel in"=w383) -> ("error out"=w380:errorcluster, "Channel out"=w382:refnum<class "Channel.lvclass">)  [unwired: 7 in]
                }
              }
            }
            frame True {
            }
          }
        }
        frame 35 {
          w396 = i16 0 items=["Cooler OFF", "Cooler ON"] ("Cooler ON/OFF")
          # "OV 2022-05-10: Ao setar a temperatura, liga \nautomaticamente o COLLER."
          n140 = Unbundle By Name(w405) -> ("Interface.lvclass"=w404:refnum<class "Interface.lvclass">)
          n141 = call-dynamic "Read Temperature.vi"("Interface in"=w404) -> ("Temperature"=w401:i8, "Interface out"=w395:refnum<class "Interface.lvclass">)  [unwired: 8 in, 1 out]
          n142 = Number To Decimal String(number=w401) -> (decimal integer string=w400:string)  [unwired: 1 in]
          n143 = Concatenate Strings("SET TEMP " ("cmd"), w400) -> (w403:string)
          n144 = call-dynamic "Write Cooler ON_OFF.vi"("Cooler ON/OFF"=w396, "Interface in"=w395) -> ("Interface out"=w394:refnum<class "Interface.lvclass">)  [unwired: 8 in, 1 out]
          n145 = call-dynamic "Write cmd.vi"("error in (no error)"=w407, "cmd"=w403, "Device in"=w405) -> ("error out"=w406:errorcluster, "Device out"=w398:refnum<class "Channel.lvclass">)  [unwired: 7 in]
          n146 = Bundle By Name(cluster=w398, "Interface.lvclass"=w394) -> (w397:refnum<class "Channel.lvclass">)
          n147 = disable-structure shown="Enabled" {
            disable-tunnel: [0 ("State") 30 ("State")] -> w399
            frame Disabled {
            }
            frame Enabled {
            }
          }
        }
        frame 50 {
          (unwired) "S4ACS C1/C2/C3/C4 EXPOSE " ("cmd")
          # "Carrega timeout de 10 ciclos\npara resposta do ACS"
          n148 = call-dynamic "Write Timer.vi"("error in (no error)"=w413, "Timer"=u32 10, "State Machine in"=w416) -> ("error out"=w412:errorcluster, "State Machine out"=w418:refnum<class "State Machine.lvclass">)  [unwired: 7 in]
          n149 = call-dynamic "Write State Machine.vi"("error in (no error)"=w412, "State Machine.lvclass"=w418, "Device in"=w415) -> ("error out"=w411:errorcluster, "Device out"=w414:refnum<class "Channel.lvclass">)  [unwired: 7 in]
          n150 = call-dynamic "Write cmd.vi"("error in (no error)"=w411, "cmd"="EXPOSE", "Device in"=w414) -> ("error out"=w421:errorcluster, "Device out"=w422:refnum<class "Channel.lvclass">)  [unwired: 7 in]
          n151 = Increment(x=w420) -> (x+1=w410:i32)
        }
        frame 51 {
          # "Verifica timeout para ACS responder.\nSe estourar timeout é porque o ACS não \nrespondeu e este canal volta para o estado 0\npara não \"travar\" os outros canais no \nS4ACS_GUI:HandleObservation.vi."
          n152 = call "Verify Timer.vi"("error in (no error)"=w427, "State Machine in"=w429) -> ("error out"=w426:errorcluster, "timeout"=w425:bool, "State Machine out"=w428:refnum<class "State Machine.lvclass">)  [unwired: 7 in]
          n153 = call-dynamic "Write State Machine.vi"("error in (no error)"=w426, "State Machine.lvclass"=w428, "Device in"=w430) -> ("error out"=w423:errorcluster, "Device out"=w424:refnum<class "Channel.lvclass">)  [unwired: 7 in]
          n154 = case shown="True" w425 {
            tunnel: [w433 w434] -> w432
            tunnel: w431 -> [w433 w435]
            frame False {
            }
            frame True {
              n155 = Increment(x=w435) -> (x+1=w434:i32)
            }
          }
        }
        frame 52 {
          (unwired) "S4ACS C1/C2/C3/C4 STATUS " ("cmd")
          # "Carrega timeout de 200 ciclos\npara resposta do ACS"
          n156 = call-dynamic "Write Timer.vi"("error in (no error)"=w439, "Timer"=u32 200, "State Machine in"=w440) -> ("error out"=w442:errorcluster, "State Machine out"=w443:refnum<class "State Machine.lvclass">)  [unwired: 7 in]
          n157 = call-dynamic "Write State Machine.vi"("error in (no error)"=w442, "State Machine.lvclass"=w443, "Device in"=w441) -> ("error out"=w438:errorcluster, "Device out"=w436:refnum<class "Channel.lvclass">)  [unwired: 7 in]
          n158 = call-dynamic "Write cmd.vi"("error in (no error)"=w438, "cmd"="STATUS", "Device in"=w436) -> ("error out"=w447:errorcluster, "Device out"=w448:refnum<class "Channel.lvclass">)  [unwired: 7 in]
          n159 = Increment(x=w445) -> (x+1=w446:i32)
        }
        frame 53 {
          # "Verifica timeout para ACS responder.\nSe estourar timeout é porque o ACS não \nrespondeu e este canal volta para o estado 0\npara não \"travar\" os outros canais no \nS4ACS_GUI:HandleObservation.vi."
          # "Status.Texp = Current frame exptime\nlastStatus = cam status (acquiring, idle, writing, reading, ...)\nStatus.Nimages = frames done"
          # "Extrair todos os parametros da respsota de STATUS e\natualizar a informação na classe Channel."
          n160 = call "Verify Timer.vi"("error in (no error)"=w449, "State Machine in"=w454) -> ("error out"=w455:errorcluster, "timeout"=w453:bool, "State Machine out"=w456:refnum<class "State Machine.lvclass">)  [unwired: 7 in]
          n161 = call-dynamic "Write State Machine.vi"("error in (no error)"=w455, "State Machine.lvclass"=w456, "Device in"=w452) -> ("error out"=w450:errorcluster, "Device out"=w451:refnum<class "Channel.lvclass">)  [unwired: 7 in]
          n162 = call-dynamic "Read resp.vi"("error in (no error)"=w450, "Device in"=w451) -> ("error out"=w478:errorcluster, "resp"=w479:string, "Device out"=w482:refnum<class "Channel.lvclass">)  [unwired: 7 in]
          "resposta do STATUS" <- w479
          n163 = call-dynamic "Read Interface.vi"("error in (no error)"=w478, "Channel in"=w482) -> ("error out"=w477:errorcluster, "Interface.lvclass"=w480:refnum<class "Interface.lvclass">, "Channel out"=w481:refnum<class "Channel.lvclass">)  [unwired: 7 in]
          n164 = call-dynamic "UpdateStatus.vi"("error in (no error)"=w477, "status"=w479, "Interface in"=w480) -> ("error out"=w462:errorcluster, "Interface out"=w465:refnum<class "Interface.lvclass">)  [unwired: 7 in]
          n165 = call-dynamic "Read Exposições realizadas.vi"("error in (no error)"=w462, "Interface in"=w465) -> ("error out"=w461:errorcluster, "Exposições realizadas"=w463:dbl, "Interface out"=w464:refnum<class "Interface.lvclass">)  [unwired: 7 in]
          n166 = call-dynamic "Read Cam_Status.vi"("error in (no error)"=w461, "Interface in"=w464) -> ("error out"=w472:errorcluster, "Cam_Status"=w457:string, "Interface out"=w474:refnum<class "Interface.lvclass">)  [unwired: 7 in]
          n167 = call-dynamic "Read %Acquired.vi"("error in (no error)"=w472, "Interface in"=w474) -> ("error out"=w471:errorcluster, "% Acquired"=w468:dbl, "Interface out"=w473:refnum<class "Interface.lvclass">)  [unwired: 7 in]
          n168 = call "Read Exposure Time.vi"("error in (no error)"=w471, "Interface in"=w473) -> ("error out"=w459:errorcluster, "Exposure Time"=w470:dbl, "Interface out"=w458:refnum<class "Interface.lvclass">)  [unwired: 7 in]
          n169 = call-dynamic "Write Interface.vi"("error in (no error)"=w459, "Interface.lvclass"=w458, "Channel in"=w481) -> ("error out"=w476:errorcluster, "Channel out"=w475:refnum<class "Channel.lvclass">)  [unwired: 7 in]
          n170 = case shown="\"ACTIVE\"" w457 {
            tunnel: [w486 w489] -> w485
            tunnel: w484 -> [w487 w490]
            tunnel: w453 -> [_ w488]
            frame "ACTIVE" {
              n171 = Increment(x=w487) -> (x+1=w486:i32)
            }
            frame Default {
              n172 = case shown="False" w488 {
                tunnel: w490 -> [w491 _]
                tunnel: [w491 0] -> w489
                frame False {
                }
                frame True {
                }
              }
            }
          }
          n173 = To Unsigned Long Integer(number=w463) -> (unsigned 32bit integer=w460:u32)
          n174 = Divide(x=w468, y=100.0) -> (x/y=w466:dbl)
          n175 = Multiply(x=w470, y=w466) -> (x*y=w469:dbl)
          n176 = Bundle By Name(cluster=w475, "Texp"=w469, "lastStatus"=w457, "Nimages"=w460) -> (w483:refnum<class "Channel.lvclass">)
        }
        frame 54 {
          # "Carrega timeout de 200 ciclos x 20ms = 4s\npara resposta do ACS"
          n177 = call-dynamic "Write Timer.vi"("error in (no error)"=w494, "Timer"=u32 200, "State Machine in"=w498) -> ("error out"=w499:errorcluster, "State Machine out"=w500:refnum<class "State Machine.lvclass">)  [unwired: 7 in]
          n178 = call-dynamic "Write State Machine.vi"("error in (no error)"=w499, "State Machine.lvclass"=w500, "Device in"=w496) -> ("error out"=w493:errorcluster, "Device out"=w495:refnum<class "Channel.lvclass">)  [unwired: 7 in]
          n179 = call-dynamic "Write cmd.vi"("error in (no error)"=w493, "cmd"="STATUS", "Device in"=w495) -> ("error out"=w504:errorcluster, "Device out"=w505:refnum<class "Channel.lvclass">)  [unwired: 7 in]
          n180 = Increment(x=w502) -> (x+1=w503:i32)
        }
        frame 55 {
          # "Status.Texp = Current frame exptime\nlastStatus = cam status (acquiring, idle, writing, reading, ...)\nStatus.Nimages = frames done"
          # "Extrair todos os parametros da respsota de STATUS e\natualizar a informação na classe Channel."
          n181 = call "Verify Timer.vi"("error in (no error)"=w511, "State Machine in"=w510) -> ("error out"=w507:errorcluster, "timeout"=w506:bool, "State Machine out"=w508:refnum<class "State Machine.lvclass">)  [unwired: 7 in]
          n182 = call-dynamic "Read resp.vi"("error in (no error)"=w507, "Device in"=w509) -> ("error out"=w535:errorcluster, "resp"=w536:string, "Device out"=w539:refnum<class "Channel.lvclass">)  [unwired: 7 in]
          n183 = call-dynamic "Read Interface.vi"("error in (no error)"=w535, "Channel in"=w539) -> ("error out"=w534:errorcluster, "Interface.lvclass"=w537:refnum<class "Interface.lvclass">, "Channel out"=w538:refnum<class "Channel.lvclass">)  [unwired: 7 in]
          n184 = call-dynamic "UpdateStatus.vi"("error in (no error)"=w534, "status"=w536, "Interface in"=w537) -> ("error out"=w521:errorcluster, "Interface out"=w524:refnum<class "Interface.lvclass">)  [unwired: 7 in]
          n185 = call-dynamic "Read Exposições realizadas.vi"("error in (no error)"=w521, "Interface in"=w524) -> ("error out"=w520:errorcluster, "Exposições realizadas"=w522:dbl, "Interface out"=w523:refnum<class "Interface.lvclass">)  [unwired: 7 in]
          n186 = call-dynamic "Read Cam_Status.vi"("error in (no error)"=w520, "Interface in"=w523) -> ("error out"=w531:errorcluster, "Cam_Status"=w516:string, "Interface out"=w533:refnum<class "Interface.lvclass">)  [unwired: 7 in]
          n187 = call-dynamic "Read %Acquired.vi"("error in (no error)"=w531, "Interface in"=w533) -> ("error out"=w530:errorcluster, "% Acquired"=w527:dbl, "Interface out"=w532:refnum<class "Interface.lvclass">)  [unwired: 7 in]
          n188 = call "Read Exposure Time.vi"("error in (no error)"=w530, "Interface in"=w532) -> ("error out"=w518:errorcluster, "Exposure Time"=w529:dbl, "Interface out"=w517:refnum<class "Interface.lvclass">)  [unwired: 7 in]
          n189 = call-dynamic "Write Interface.vi"("error in (no error)"=w518, "Interface.lvclass"=w517, "Channel in"=w538) -> ("error out"=w515:errorcluster, "Channel out"=w514:refnum<class "Channel.lvclass">)  [unwired: 7 in]
          n190 = case shown="Default" w516 {
            tunnel: [32 ("State") w558 w572] -> w542
            tunnel: w541 -> [_ w559 w573]
            tunnel: w515 -> [w549 w554 w570]
            tunnel: [w546 w556 w567] -> w513
            tunnel: w514 -> [w547 w557 w571]
            tunnel: [w543 w553 w564] -> w512
            tunnel: w508 -> [w550 w555 w569]
            tunnel: w506 -> [_ w552 w563]
            frame "ACQUISITION ABORTED", "IDLE" {
              # "250x20ms=5s"
              n191 = call-dynamic "Write Timer.vi"("error in (no error)"=w549, "Timer"=u32 250, "State Machine in"=w550) -> ("error out"=w544:errorcluster, "State Machine out"=w545:refnum<class "State Machine.lvclass">)  [unwired: 7 in]
              n192 = call-dynamic "Write State Machine.vi"("error in (no error)"=w544, "State Machine.lvclass"=w545, "Device in"=w547) -> ("error out"=w543:errorcluster, "Device out"=w546:refnum<class "Channel.lvclass">)  [unwired: 7 in]
            }
            frame Default {
              n193 = case shown="False" w552 {
                tunnel: w559 -> [w561 _]
                tunnel: [w560 0] -> w558
                frame False {
                  n194 = Decrement(x=w561) -> (x-1=w560:i32)
                }
                frame True {
                }
              }
              n195 = call-dynamic "Write State Machine.vi"("error in (no error)"=w554, "State Machine.lvclass"=w555, "Device in"=w557) -> ("error out"=w553:errorcluster, "Device out"=w556:refnum<class "Channel.lvclass">)  [unwired: 7 in]
            }
            frame "" {
              # "STATUS=\"\"\nACS parado"
              n196 = case shown="False" w563 {
                tunnel: w573 -> [w574 _]
                tunnel: [w574 0] -> w572
                tunnel: w571 -> [w577 w580]
                tunnel: [w577 w580] -> w568
                tunnel: w570 -> [w576 w581]
                tunnel: [w576 w578] -> w565
                tunnel: w569 -> [w575 w583]
                tunnel: [w575 w579] -> w566
                frame False {
                }
                frame True {
                  n197 = call-dynamic "Write Timer.vi"("error in (no error)"=w581, "Timer"=u32 250, "State Machine in"=w583) -> ("error out"=w578:errorcluster, "State Machine out"=w579:refnum<class "State Machine.lvclass">)  [unwired: 7 in]
                }
              }
              n198 = call-dynamic "Write State Machine.vi"("error in (no error)"=w565, "State Machine.lvclass"=w566, "Device in"=w568) -> ("error out"=w564:errorcluster, "Device out"=w567:refnum<class "Channel.lvclass">)  [unwired: 7 in]
            }
          }
          n199 = To Unsigned Long Integer(number=w522) -> (unsigned 32bit integer=w519:u32)
          n200 = Divide(x=w527, y=100.0) -> (x/y=w525:dbl)
          n201 = Multiply(x=w529, y=w525) -> (x*y=w528:dbl)
          n202 = Bundle By Name(cluster=w513, "Texp"=w528, "lastStatus"=w516, "Nimages"=w519) -> (w540:refnum<class "Channel.lvclass">)
        }
        frame 56 {
          # "Pedido de STATUS para verificar conexão com ACS"
          # "Carrega timeout de 10 ciclos \n(20 x 20ms = 0.4s) \npara resposta do ACS"
          n203 = call-dynamic "Write Timer.vi"("error in (no error)"=w590, "Timer"=u32 20, "State Machine in"=w594) -> ("error out"=w595:errorcluster, "State Machine out"=w596:refnum<class "State Machine.lvclass">)  [unwired: 7 in]
          n204 = call-dynamic "Write State Machine.vi"("error in (no error)"=w595, "State Machine.lvclass"=w596, "Device in"=w592) -> ("error out"=w589:errorcluster, "Device out"=w591:refnum<class "Channel.lvclass">)  [unwired: 7 in]
          n205 = call-dynamic "Write cmd.vi"("error in (no error)"=w589, "cmd"="STATUS", "Device in"=w591) -> ("error out"=w587:errorcluster, "Device out"=w588:refnum<class "Channel.lvclass">)  [unwired: 7 in]
          n206 = Increment(x=w598) -> (x+1=w599:i32)
          n207 = disable-structure shown="Enabled" {
            disable-tunnel: w588 -> [w604 w606]
            disable-tunnel: w587 -> [w603 w605]
            disable-tunnel: [w602 w605] -> w586
            disable-tunnel: [w601 w606] -> w585
            frame Enabled {
              n208 = call "Write connected.vi"("error in (no error)"=w603, "connected"=FALSE, "Device in"=w604) -> ("error out"=w602:errorcluster, "Device out"=w601:refnum<class "Channel.lvclass">)  [unwired: 7 in]
            }
            frame Disabled {
            }
          }
        }
        frame 57 {
          # "Status.Texp = Current frame exptime\nlastStatus = cam status (acquiring, idle, writing, reading, ...)\nStatus.Nimages = frames done"
          # "Extrair todos os parametros da respsota de STATUS e\natualizar a informação na classe Channel."
          n209 = call "Verify Timer.vi"("error in (no error)"=w617, "State Machine in"=w616) -> ("error out"=w613:errorcluster, "State Machine out"=w615:refnum<class "State Machine.lvclass">)  [unwired: 7 in, 1 out]
          n210 = call-dynamic "Read Timeout.vi"("error in (no error)"=w613, "State Machine in"=w615) -> ("error out"=w608:errorcluster, "Timeout"=w612:bool, "State Machine out"=w614:refnum<class "State Machine.lvclass">)  [unwired: 7 in]
          n211 = call "Read connected.vi"("error in (no error)"=w608, "Device in"=w611) -> ("error out"=w609:errorcluster, "connected"=w607:bool, "Device out"=w610:refnum<class "Channel.lvclass">)  [unwired: 7 in]
          n212 = call-dynamic "Read resp.vi"("error in (no error)"=w609, "Device in"=w610) -> ("error out"=w641:errorcluster, "resp"=w642:string, "Device out"=w645:refnum<class "Channel.lvclass">)  [unwired: 7 in]
          n213 = call-dynamic "Read Interface.vi"("error in (no error)"=w641, "Channel in"=w645) -> ("error out"=w640:errorcluster, "Interface.lvclass"=w643:refnum<class "Interface.lvclass">, "Channel out"=w644:refnum<class "Channel.lvclass">)  [unwired: 7 in]
          n214 = call-dynamic "UpdateStatus.vi"("error in (no error)"=w640, "status"=w642, "Interface in"=w643) -> ("error out"=w627:errorcluster, "Interface out"=w630:refnum<class "Interface.lvclass">)  [unwired: 7 in]
          n215 = call-dynamic "Read Exposições realizadas.vi"("error in (no error)"=w627, "Interface in"=w630) -> ("error out"=w626:errorcluster, "Exposições realizadas"=w628:dbl, "Interface out"=w629:refnum<class "Interface.lvclass">)  [unwired: 7 in]
          n216 = call-dynamic "Read Cam_Status.vi"("error in (no error)"=w626, "Interface in"=w629) -> ("error out"=w637:errorcluster, "Cam_Status"=w622:string, "Interface out"=w639:refnum<class "Interface.lvclass">)  [unwired: 7 in]
          n217 = call-dynamic "Read %Acquired.vi"("error in (no error)"=w637, "Interface in"=w639) -> ("error out"=w636:errorcluster, "% Acquired"=w633:dbl, "Interface out"=w638:refnum<class "Interface.lvclass">)  [unwired: 7 in]
          n218 = call "Read Exposure Time.vi"("error in (no error)"=w636, "Interface in"=w638) -> ("error out"=w624:errorcluster, "Exposure Time"=w635:dbl, "Interface out"=w623:refnum<class "Interface.lvclass">)  [unwired: 7 in]
          n219 = call-dynamic "Write Interface.vi"("error in (no error)"=w624, "Interface.lvclass"=w623, "Channel in"=w644) -> ("error out"=w621:errorcluster, "Channel out"=w620:refnum<class "Channel.lvclass">)  [unwired: 7 in]
          n220 = case shown="True" w607 {
            tunnel: [w651 w668] -> w648
            tunnel: w647 -> [w652 w669]
            tunnel: w621 -> [w649 w666]
            tunnel: [w654 w663] -> w619
            tunnel: w620 -> [w655 w667]
            tunnel: [w653 w660] -> w618
            tunnel: w614 -> [w650 w665]
            tunnel: w612 -> [_ w659]
            frame True {
              # "Conneted=T\nACS respondeu"
              n221 = disable-structure shown="Enabled" {
                disable-tunnel: w652 -> [w657 _]
                disable-tunnel: [w656 0] -> w651
                frame Enabled {
                  n222 = Increment(x=w657) -> (x+1=w656:i32)
                }
                frame Disabled {
                }
              }
              n223 = call-dynamic "Write State Machine.vi"("error in (no error)"=w649, "State Machine.lvclass"=w650, "Device in"=w655) -> ("error out"=w653:errorcluster, "Device out"=w654:refnum<class "Channel.lvclass">)  [unwired: 7 in]
            }
            frame False {
              # "Conneted=F\nACS não resp."
              n224 = case shown="False" w659 {
                tunnel: w669 -> [w670 _]
                tunnel: [w670 0] -> w668
                tunnel: w667 -> [w673 w676]
                tunnel: [w673 w676] -> w664
                tunnel: w666 -> [w672 w677]
                tunnel: [w672 w674] -> w661
                tunnel: w665 -> [w671 w679]
                tunnel: [w671 w675] -> w662
                frame False {
                }
                frame True {
                  n225 = call-dynamic "Write Timer.vi"("error in (no error)"=w677, "Timer"=u32 250, "State Machine in"=w679) -> ("error out"=w674:errorcluster, "State Machine out"=w675:refnum<class "State Machine.lvclass">)  [unwired: 7 in]
                }
              }
              n226 = call-dynamic "Write State Machine.vi"("error in (no error)"=w661, "State Machine.lvclass"=w662, "Device in"=w664) -> ("error out"=w660:errorcluster, "Device out"=w663:refnum<class "Channel.lvclass">)  [unwired: 7 in]
            }
          }
          n227 = Divide(x=w633, y=100.0) -> (x/y=w631:dbl)
          n228 = To Unsigned Long Integer(number=w628) -> (unsigned 32bit integer=w625:u32)
          n229 = Multiply(x=w635, y=w631) -> (x*y=w634:dbl)
          n230 = Bundle By Name(cluster=w619, "Texp"=w634, "lastStatus"=w622, "Nimages"=w625) -> (w646:refnum<class "Channel.lvclass">)
        }
        frame 58 {
          (unwired) " \r" ("regular expression")
          w686 = "HUM=" ("regular expression")
          # "Passa valores da telemetria adquiridos do TCS"
          n231 = call-dynamic "Write State Machine.vi"("error in (no error)"=w681, "State Machine.lvclass"=w682, "Device in"=w693) -> ("error out"=w690:errorcluster, "Device out"=w692:refnum<class "Channel.lvclass">)  [unwired: 7 in]
          n232 = Unbundle By Name(w692) -> ("TCS telemetry"=w687:string, "Filter"=w689:u8)
          n233 = Match Pattern(string=w687, regular expression=w686) -> (before substring=w685:string, match substring=w684:string, after substring=w683:string)  [unwired: 1 in, 1 out]
          n234 = Equal?(x=w684, y=w686) -> (x = y?=w688:bool)
          n235 = case shown="True" w688 {
            tunnel: [w697 w714] -> w695
            tunnel: [w696 w713] -> w694
            tunnel: w692 -> [w697 w712]
            tunnel: w690 -> [w696 w706]
            tunnel: w689 -> [_ w705]
            tunnel: w685 -> [_ w701]
            tunnel: w684 -> [_ w700]
            tunnel: w683 -> [_ w699]
            frame False {
            }
            frame True {
              w702 = " \r" ("regular expression")
              n236 = case shown="0, Default" w705 {
                tunnel: ["CLEAR" ("string") "U" ("string") "B" ("string") "V" ("string") "R" ("string") "I" ("string")] -> w704
                frame 0, Default {
                }
                frame 1 {
                }
                frame 2 {
                }
                frame 3 {
                }
                frame 4 {
                }
                frame 5 {
                }
              }
              n237 = call <vilib>:"Trim Whitespace.vi"("string"=w699) -> ("trimmed string"=w698:string)  [unwired: 1 in]
              n238 = disable-structure shown="Enabled" {
                disable-tunnel: [w717 w718] -> w708
                disable-tunnel: w701 -> [w716 w721]
                disable-tunnel: w702 -> [w715 _]
                disable-tunnel: w700 -> [_ w720]
                disable-tunnel: w698 -> [_ w719]
                frame Disabled {
                  n239 = Match Pattern(string=w716, regular expression=w715) -> (before substring=w717:string)  [unwired: 1 in, 3 out]
                }
                frame Enabled {
                  n240 = Concatenate Strings(w721, w720, w719) -> (w718:string)
                }
              }
              n241 = Concatenate Strings(w708, " FILTER=" ("string"), w704, " CTRLINTE=S4GUI" ("string"), w702) -> (w707:string)
              n242 = Concatenate Strings("WRITE_TCS_DATA " ("cmd"), w707) -> (w710:string)
              n243 = call-dynamic "Write cmd.vi"("error in (no error)"=w706, "cmd"=w710, "Device in"=w712) -> ("error out"=w713:errorcluster, "Device out"=w714:refnum<class "Channel.lvclass">)  [unwired: 7 in]
            }
          }
        }
        frame 60 {
          # "Carrega timeout de 5 ciclos\npara resposta do ACS"
          n244 = call-dynamic "Write Timer.vi"("Timer"=u32 5, "State Machine in"=w733) -> ("error out"=w734:errorcluster, "State Machine out"=w732:refnum<class "State Machine.lvclass">)  [unwired: 8 in]
          n245 = call-dynamic "Write State Machine.vi"("error in (no error)"=w734, "State Machine.lvclass"=w732, "Device in"=w731) -> ("Device out"=w730:refnum<class "Channel.lvclass">)  [unwired: 7 in, 1 out]
          n246 = disable-structure shown="Enabled" {
            disable-tunnel: [w745 w747] -> w738
            disable-tunnel: w737 -> [w744 w746]
            disable-tunnel: [w743 w746] -> w736
            disable-tunnel: w730 -> [w741 w747]
            disable-tunnel: w729 -> [w740 _]
            disable-tunnel: [w739 62] -> w728
            frame Disabled {
              n247 = Increment(x=w740) -> (x+1=w739:i32)
              n248 = call-dynamic "Write cmd.vi"("error in (no error)"=w744, "cmd"="INIT", "Device in"=w741) -> ("error out"=w743:errorcluster, "Device out"=w745:refnum<class "Channel.lvclass">)  [unwired: 7 in]
            }
            frame Enabled {
            }
          }
        }
        frame 61 {
          w758 = "INITIALIZATION"
          # "Verifica timeout para ACS responder.\nSe estourar timeout é porque o ACS não \nrespondeu e este canal volta para o estado 0\npara não \"travar\" os outros canais no \nS4ACS_GUI:HandleObservation.vi."
          n249 = call "Verify Timer.vi"("error in (no error)"=w749, "State Machine in"=w754) -> ("error out"=w755:errorcluster, "timeout"=w750:bool, "State Machine out"=w756:refnum<class "State Machine.lvclass">)  [unwired: 7 in]
          n250 = call-dynamic "Write State Machine.vi"("error in (no error)"=w755, "State Machine.lvclass"=w756, "Device in"=w753) -> ("error out"=w751:errorcluster, "Device out"=w752:refnum<class "Channel.lvclass">)  [unwired: 7 in]
          n251 = call-dynamic "Read resp.vi"("error in (no error)"=w751, "Device in"=w752) -> ("error out"=w762:errorcluster, "resp"=w760:string, "Device out"=w763:refnum<class "Channel.lvclass">)  [unwired: 7 in]
          "resp INIT" <- w760
          n252 = Match Pattern(string=w760, regular expression=w758) -> (match substring=w759:string)  [unwired: 1 in, 3 out]
          n253 = Equal?(x=w759, y=w758) -> (x = y?=w757:bool)
          n254 = case shown="True" w757 {
            tunnel: [w765 w770] -> w764
            tunnel: w761 -> [w766 w771]
            tunnel: w750 -> [w767 _]
            frame False {
              n255 = case shown="True" w767 {
                tunnel: [w768 0 ("State")] -> w765
                tunnel: w766 -> [w768 _]
                frame False {
                }
                frame True {
                }
              }
            }
            frame True {
              n256 = disable-structure shown="Enabled" {
                disable-tunnel: w771 -> [w773 _]
                disable-tunnel: [w772 54] -> w770
                frame Disabled {
                  n257 = Increment(x=w773) -> (x+1=w772:i32)
                }
                frame Enabled {
                  # "debug:\nNão deve enviar\n WRITE_SETUP para o \nACS antigo"
                }
              }
            }
          }
        }
        frame 62 {
          # "Carrega timeout de 50 ciclos\npara resposta do ACS"
          n258 = call-dynamic "Write Timer.vi"("error in (no error)"=w784, "Timer"=u32 50, "State Machine in"=w787) -> ("error out"=w788:errorcluster, "State Machine out"=w786:refnum<class "State Machine.lvclass">)  [unwired: 7 in]
          n259 = call-dynamic "Write State Machine.vi"("error in (no error)"=w788, "State Machine.lvclass"=w786, "Device in"=w785) -> ("error out"=w781:errorcluster, "Device out"=w783:refnum<class "Channel.lvclass">)  [unwired: 7 in]
          n260 = Unbundle By Name(w783) -> ("Interface.lvclass"=w782:refnum<class "Interface.lvclass">)
          n261 = call-dynamic "Get CCD_Config.vi"("error in (no error)"=w781, "Interface in"=w782) -> ("error out"=w776:errorcluster, "output cluster"=w778:T2)  [unwired: 7 in, 1 out]
          n262 = Flatten To JSON(anything=w778, error in (no error)=w776) -> (JSON string=w777:string, 11:w775:errorcluster)  [unwired: 1 in]
          n263 = Concatenate Strings("WRITE_SETUP " ("cmd"), w777) -> (w779:string)
          n264 = call-dynamic "Write cmd.vi"("error in (no error)"=w775, "cmd"=w779, "Device in"=w783) -> ("error out"=w792:errorcluster, "Device out"=w793:refnum<class "Channel.lvclass">)  [unwired: 7 in]
          n265 = Increment(x=w790) -> (x+1=w791:i32)
        }
        frame 63 {
          # "Não há resposta para o comando WRTITE_SETUP\nQuando estourar timeout vai para o estado 54 para \nobter o STATUS do ACS."
          n266 = call "Verify Timer.vi"("error in (no error)"=w797, "State Machine in"=w799) -> ("error out"=w800:errorcluster, "timeout"=w796:bool, "State Machine out"=w801:refnum<class "State Machine.lvclass">)  [unwired: 7 in]
          n267 = call-dynamic "Write State Machine.vi"("error in (no error)"=w800, "State Machine.lvclass"=w801, "Device in"=w798) -> ("error out"=w794:errorcluster, "Device out"=w795:refnum<class "Channel.lvclass">)  [unwired: 7 in]
          n268 = case shown="True" w796 {
            tunnel: [w804 w805] -> w803
            tunnel: w802 -> [w804 w806]
            frame False {
            }
            frame True {
              n269 = Increment(x=w806) -> (x+1=w805:i32)
            }
          }
        }
        frame 64 {
          # "Carrega timeout de 50 ciclos\npara resposta do ACS"
          n270 = call-dynamic "Write Timer.vi"("error in (no error)"=w810, "Timer"=u32 50, "State Machine in"=w813) -> ("error out"=w814:errorcluster, "State Machine out"=w812:refnum<class "State Machine.lvclass">)  [unwired: 7 in]
          n271 = call-dynamic "Write State Machine.vi"("error in (no error)"=w814, "State Machine.lvclass"=w812, "Device in"=w811) -> ("error out"=w807:errorcluster, "Device out"=w809:refnum<class "Channel.lvclass">)  [unwired: 7 in]
          n272 = call-dynamic "Write cmd.vi"("error in (no error)"=w807, "cmd"="READ_SETUP ", "Device in"=w809) -> ("error out"=w818:errorcluster, "Device out"=w819:refnum<class "Channel.lvclass">)  [unwired: 7 in]
          n273 = Increment(x=w816) -> (x+1=w817:i32)
        }
        frame 65 {
          n274 = call "Verify Timer.vi"("error in (no error)"=w841, "State Machine in"=w843) -> ("error out"=w844:errorcluster, "timeout"=w829:bool, "State Machine out"=w845:refnum<class "State Machine.lvclass">)  [unwired: 7 in]
          n275 = call-dynamic "Write State Machine.vi"("error in (no error)"=w844, "State Machine.lvclass"=w845, "Device in"=w842) -> ("error out"=w839:errorcluster, "Device out"=w840:refnum<class "Channel.lvclass">)  [unwired: 7 in]
          n276 = call-dynamic "Read resp.vi"("error in (no error)"=w839, "Device in"=w840) -> ("error out"=w833:errorcluster, "resp"=w831:string, "Device out"=w838:refnum<class "Channel.lvclass">)  [unwired: 7 in]
          n277 = Unbundle By Name(w838) -> ("Interface.lvclass"=w834:refnum<class "Interface.lvclass">)
          n278 = call-dynamic "Get CCD_Config.vi"("error in (no error)"=w833, "Interface in"=w834) -> ("error out"=w835:errorcluster, "output cluster"=w832:T2, "Interface out"=w836:refnum<class "Interface.lvclass">)  [unwired: 7 in]
          n279 = String Length(string=w831) -> (length=w830:i32)
          n280 = Greater Than 0?(x=w830) -> (x > 0?=w825:bool)
          n281 = case shown="True" w825 {
            tunnel: w836 -> [w849 w855]
            tunnel: w835 -> [w848 w854]
            tunnel: w832 -> [_ w858]
            tunnel: w831 -> [_ w857]
            tunnel: [w849 w853] -> w823
            tunnel: [w848 w852] -> w824
            tunnel: [T1 {"ACQUISITION_MODE"=FALSE, "TRIGGER_MODE"=FALSE, "READ_MODE"=FALSE, "PREAMP"=FALSE, "READOUT_RATE"=FALSE, "VERTICAL_SHIFT_SPEED"=FALSE, "EM_MODE"=FALSE, "EM_GAIN"=FALSE, "SHUTTER_MODE"=FALSE, "SHUTTER_TTL"=FALSE, "SHUTTER_OPENING_TIME"=FALSE, "SHUTTER_CLOSING_TIME"=FALSE, "VBIN"=FALSE, "HBIN"=FALSE, "INITIAL_LINE"=FALSE, "INITIAL_COLUMN"=FALSE, "FINAL_LINE"=FALSE, "FINAL_COLUMN"=FALSE, "FRAME_TRANSFER"=FALSE, "VERTICAL_CLOCK_VOLTAGE"=FALSE, "AD_CHANNEL"=FALSE} ("x = y?") w856] -> w822
            frame False {
            }
            frame True {
              n282 = Unflatten From JSON(JSON string=w857, type and defaults=w858) -> (value=w851:T2)  [unwired: 5 in, 1 out]
              n283 = Equal?(x=w851, y=w858) -> (x = y?=w856:T1)
              n284 = call-dynamic "Set CCD_Config.vi"("error in (no error)"=w854, "input cluster"=w851, "Interface in"=w855) -> ("error out"=w852:errorcluster, "Interface out"=w853:refnum<class "Interface.lvclass">)  [unwired: 7 in]
            }
          }
          "x = y?" <- w822
          n285 = Or(x=w829, y=w825) -> (x .or. y?=w828:bool)
          n286 = call "Write Checked Params.vi"("error in (no error)"=w824, "Checked Params"=w822, "Interface in"=w823) -> ("error out"=w820:errorcluster, "Interface out"=w821:refnum<class "Interface.lvclass">)  [unwired: 7 in]
          n287 = case shown="False" w828 {
            tunnel: [w861 w865] -> w847
            tunnel: w846 -> [w861 w862]
            tunnel: w821 -> [w860 w863]
            tunnel: [w860 w863] -> w827
            tunnel: w820 -> [w859 w864]
            tunnel: [w859 w864] -> w826
            frame False {
            }
            frame True {
              n288 = disable-structure shown="Enabled" {
                disable-tunnel: [54 ("State") w867] -> w865
                disable-tunnel: w862 -> [_ w868]
                frame Disabled {
                }
                frame Enabled {
                  n289 = Increment(x=w868) -> (x+1=w867:i32)
                }
              }
            }
          }
          n290 = Bundle By Name(cluster=w838, "Interface.lvclass"=w827) -> (w837:refnum<class "Channel.lvclass">)
        }
        frame 66 {
          # "O valor do COOLER aqui\nfoi carregado no Acquistion:Init.vi"
          # "Se COOLER=0\n        SET COLLERPOWER_STATUS 0\n        AVANÇA ESTADO\n        VAI PRA 0\nSe COOLER=1:\n      DESVIA PARA Estado 35"
          # "Carrega timeout de 50 ciclos\npara resposta do ACS"
          n291 = call-dynamic "Write Timer.vi"("error in (no error)"=w876, "Timer"=u32 50, "State Machine in"=w877) -> ("error out"=w874:errorcluster, "State Machine out"=w873:refnum<class "State Machine.lvclass">)  [unwired: 7 in]
          n292 = call-dynamic "Write State Machine.vi"("error in (no error)"=w874, "State Machine.lvclass"=w873, "Device in"=w875) -> ("error out"=w872:errorcluster, "Device out"=w871:refnum<class "Channel.lvclass">)  [unwired: 7 in]
          n293 = Unbundle By Name(w871) -> ("Interface.lvclass"=w870:refnum<class "Interface.lvclass">)
          n294 = call-dynamic "Read Cooler ON_OFF.vi"("Interface in"=w870) -> ("Cooler ON/OFF"=w869:i16)  [unwired: 8 in, 2 out]
          n295 = case shown="1" w869 {
            tunnel: [w885 w892] -> w882
            tunnel: [w884 w891] -> w881
            tunnel: [35 w890] -> w880
            tunnel: w879 -> [_ w889]
            tunnel: w872 -> [w884 w887]
            tunnel: w871 -> [w885 w886]
            frame 1 {
              # "Se COOLER foi carregado com 1 na inicialização.\ndesvia para 35 para setar a temperatura e ligar o COOLER."
            }
            frame 0, Default {
              n296 = Increment(x=w889) -> (x+1=w890:i32)
              n297 = call-dynamic "Write cmd.vi"("error in (no error)"=w887, "cmd"="SET COOLER_POWER_STATUS 0", "Device in"=w886) -> ("error out"=w891:errorcluster, "Device out"=w892:refnum<class "Channel.lvclass">)  [unwired: 7 in]
            }
          }
        }
        frame 67 {
          n298 = call "Verify Timer.vi"("error in (no error)"=w896, "State Machine in"=w900) -> ("error out"=w895:errorcluster, "timeout"=w893:bool, "State Machine out"=w897:refnum<class "State Machine.lvclass">)  [unwired: 7 in]
          n299 = call-dynamic "Write State Machine.vi"("error in (no error)"=w895, "State Machine.lvclass"=w897, "Device in"=w899) -> ("error out"=w894:errorcluster, "Device out"=w898:refnum<class "Channel.lvclass">)  [unwired: 7 in]
          n300 = call-dynamic "Read resp.vi"("error in (no error)"=w894, "Device in"=w898) -> ("error out"=w902:errorcluster, "resp"=w907:string, "Device out"=w903:refnum<class "Channel.lvclass">)  [unwired: 7 in]
          n301 = Equal?(x=w907, y="DONE") -> (x = y?=w905:bool)
          n302 = case shown="True" w905 {
            tunnel: [w908 w913] -> w904
            tunnel: w901 -> [w909 _]
            tunnel: w893 -> [w910 _]
            frame False {
              n303 = case shown="False" w910 {
                tunnel: [w911 0 ("State")] -> w908
                tunnel: w909 -> [w911 _]
                frame False {
                }
                frame True {
                }
              }
            }
            frame True {
              n304 = disable-structure shown="Enabled" {
                disable-tunnel: [54 ("State") 32 ("State")] -> w913
                frame Disabled {
                }
                frame Enabled {
                  # "Lê COOLER e \nvai pra 0."
                }
              }
            }
          }
        }
        frame 70 {
          # "Carrega timeout de 5 ciclos\npara resposta do ACS"
          n305 = call-dynamic "Write Timer.vi"("error in (no error)"=w918, "Timer"=u32 5, "State Machine in"=w920) -> ("error out"=w922:errorcluster, "State Machine out"=w921:refnum<class "State Machine.lvclass">)  [unwired: 7 in]
          n306 = call-dynamic "Write State Machine.vi"("error in (no error)"=w922, "State Machine.lvclass"=w921, "Device in"=w919) -> ("error out"=w917:errorcluster, "Device out"=w916:refnum<class "Channel.lvclass">)  [unwired: 7 in]
          n307 = call-dynamic "Write cmd.vi"("error in (no error)"=w917, "cmd"="STOP_ACQUISITION", "Device in"=w916) -> ("error out"=w927:errorcluster, "Device out"=w928:refnum<class "Channel.lvclass">)  [unwired: 7 in]
          n308 = Increment(x=w925) -> (x+1=w926:i32)
        }
        frame 71 {
          w930 = "DONE"
          n309 = call-dynamic "Read resp.vi"("error in (no error)"=w937, "Device in"=w938) -> ("error out"=w934:errorcluster, "resp"=w932:string, "Device out"=w935:refnum<class "Channel.lvclass">)  [unwired: 7 in]
          "resp STOP" <- w932
          n310 = Match Pattern(string=w932, regular expression=w930) -> (match substring=w931:string)  [unwired: 1 in, 3 out]
          n311 = Equal?(x=w931, y=w930) -> ()  [unwired: 1 out]
          n312 = case shown="True" TRUE {
            tunnel: [w939 52 ("State")] -> w936
            tunnel: w933 -> [w939 _]
            frame False {
            }
            frame True {
            }
          }
        }
        frame 80 {
          n313 = call-dynamic "Write cmd.vi"("error in (no error)"=w946, "cmd"="ABORT_ACQUISITION", "Device in"=w944) -> ("error out"=w945:errorcluster, "Device out"=w947:refnum<class "Channel.lvclass">)  [unwired: 7 in]
          n314 = Increment(x=w942) -> (x+1=w943:i32)
        }
        frame 81 {
          w949 = "DONE"
          n315 = call-dynamic "Read resp.vi"("error in (no error)"=w956, "Device in"=w957) -> ("error out"=w953:errorcluster, "resp"=w951:string, "Device out"=w954:refnum<class "Channel.lvclass">)  [unwired: 7 in]
          "resp ABORT" <- w951
          n316 = Match Pattern(string=w951, regular expression=w949) -> (match substring=w950:string)  [unwired: 1 in, 3 out]
          n317 = Equal?(x=w950, y=w949) -> ()  [unwired: 1 out]
          n318 = case shown="True" TRUE {
            tunnel: [w958 52 ("State")] -> w955
            tunnel: w952 -> [w958 _]
            frame False {
            }
            frame True {
            }
          }
        }
        frame 100 {
          (unwired) "S4ACS C1/C2/C3/C4 NIMAGES " ("cmd")
          n319 = call-dynamic "Write cmd.vi"("error in (no error)"=w965, "cmd"="INIT", "Device in"=w963) -> ("error out"=w964:errorcluster, "Device out"=w966:refnum<class "Channel.lvclass">)  [unwired: 7 in]
          n320 = Increment(x=w961) -> (x+1=w962:i32)
        }
        frame 101 {
          w968 = "\r\n"
          n321 = call-dynamic "Read resp.vi"("error in (no error)"=w976, "Device in"=w977) -> ("error out"=w973:errorcluster, "resp"=w967:string, "Device out"=w970:refnum<class "Channel.lvclass">)  [unwired: 7 in]
          n322 = Match Pattern(string=w967, regular expression=w968) -> (match substring=w971:string)  [unwired: 1 in, 3 out]
          n323 = Equal?(x=w971, y=w968) -> (x = y?=w975:bool)
          n324 = case shown="False" w975 {
            tunnel: [w978 u8 0] -> w974
            tunnel: w972 -> [w978 _]
            tunnel: w970 -> [w979 w983]
            tunnel: [w979 w982] -> w969
            tunnel: w967 -> [_ w981]
            frame False {
            }
            frame True {
              n325 = Bundle By Name(cluster=w983, "lastStatus"=w981) -> (w982:refnum<class "Channel.lvclass">)
            }
          }
        }
        frame 102 {
          w991 = "EXPTIME "
          n326 = Unbundle By Name(w985) -> ("lastStatus"=w986:string)
          n327 = Match Pattern(string=w986, regular expression=w991) -> (match substring=w990:string, after substring=w988:string)  [unwired: 1 in, 2 out]
          n328 = Equal?(x=w990, y=w991) -> (x = y?=w994:bool)
          n329 = case shown="True" w994 {
            tunnel: [w995 w997] -> w993
            tunnel: w992 -> [w995 w997]
            tunnel: w985 -> [w996 w1003]
            tunnel: [w996 w1001] -> w989
            tunnel: w988 -> [_ w999]
            frame False {
            }
            frame True {
              n330 = call <vilib>:"Space Constant.vi"() -> ("String"=w1000:string)
              n331 = Match Pattern(string=w999, regular expression=w1000) -> (before substring=w998:string)  [unwired: 1 in, 3 out]
              n332 = Fract/Exp String To Number(string=w998) -> (number=w1002:dbl)  [unwired: 3 in, 1 out]
              n333 = Bundle By Name(cluster=w1003, "Texp"=w1002) -> (w1001:refnum<class "Channel.lvclass">)
            }
          }
          n334 = Increment(x=w993) -> (x+1=w984:i32)
        }
        frame 103 {
          w1011 = "NIMAGES "
          n335 = Unbundle By Name(w1005) -> ("lastStatus"=w1006:string)
          n336 = Match Pattern(string=w1006, regular expression=w1011) -> (match substring=w1010:string, after substring=w1008:string)  [unwired: 1 in, 2 out]
          n337 = Equal?(x=w1010, y=w1011) -> (x = y?=w1014:bool)
          n338 = case shown="True" w1014 {
            tunnel: [w1015 w1017] -> w1013
            tunnel: w1012 -> [w1015 w1017]
            tunnel: w1005 -> [w1016 w1023]
            tunnel: [w1016 w1021] -> w1009
            tunnel: w1008 -> [_ w1019]
            frame False {
            }
            frame True {
              n339 = call <vilib>:"Space Constant.vi"() -> ("String"=w1020:string)
              n340 = Match Pattern(string=w1019, regular expression=w1020) -> (before substring=w1018:string)  [unwired: 1 in, 3 out]
              n341 = Fract/Exp String To Number(string=w1018) -> (number=w1022:dbl)  [unwired: 3 in, 1 out]
              n342 = Bundle By Name(cluster=w1023, "Nimages"=w1022) -> (w1021:refnum<class "Channel.lvclass">)
            }
          }
          n343 = Increment(x=w1013) -> (x+1=w1004:i32)
        }
        frame 104 {
          w1031 = "INITIAL_LINE "
          n344 = Unbundle By Name(w1025) -> ("lastStatus"=w1026:string)
          n345 = Match Pattern(string=w1026, regular expression=w1031) -> (match substring=w1030:string, after substring=w1028:string)  [unwired: 1 in, 2 out]
          n346 = Equal?(x=w1030, y=w1031) -> (x = y?=w1034:bool)
          n347 = case shown="True" w1034 {
            tunnel: [w1035 w1037] -> w1033
            tunnel: w1032 -> [w1035 w1037]
            tunnel: w1025 -> [w1036 w1043]
            tunnel: [w1036 w1041] -> w1029
            tunnel: w1028 -> [_ w1039]
            frame False {
            }
            frame True {
              n348 = call <vilib>:"Space Constant.vi"() -> ("String"=w1040:string)
              n349 = Match Pattern(string=w1039, regular expression=w1040) -> (before substring=w1038:string)  [unwired: 1 in, 3 out]
              n350 = Fract/Exp String To Number(string=w1038) -> (number=w1042:dbl)  [unwired: 3 in, 1 out]
              n351 = Bundle By Name(cluster=w1043, "InitialLine"=w1042) -> (w1041:refnum<class "Channel.lvclass">)
            }
          }
          n352 = Increment(x=w1033) -> (x+1=w1024:i32)
        }
        frame 105 {
          w1051 = "FINAL_LINE "
          n353 = Unbundle By Name(w1045) -> ("lastStatus"=w1046:string)
          n354 = Match Pattern(string=w1046, regular expression=w1051) -> (match substring=w1050:string, after substring=w1048:string)  [unwired: 1 in, 2 out]
          n355 = Equal?(x=w1050, y=w1051) -> (x = y?=w1054:bool)
          n356 = case shown="True" w1054 {
            tunnel: [w1055 w1057] -> w1053
            tunnel: w1052 -> [w1055 w1057]
            tunnel: w1045 -> [w1056 w1063]
            tunnel: [w1056 w1061] -> w1049
            tunnel: w1048 -> [_ w1059]
            frame False {
            }
            frame True {
              n357 = call <vilib>:"Space Constant.vi"() -> ("String"=w1060:string)
              n358 = Match Pattern(string=w1059, regular expression=w1060) -> (before substring=w1058:string)  [unwired: 1 in, 3 out]
              n359 = Fract/Exp String To Number(string=w1058) -> (number=w1062:dbl)  [unwired: 3 in, 1 out]
              n360 = Bundle By Name(cluster=w1063, "FinalLine"=w1062) -> (w1061:refnum<class "Channel.lvclass">)
            }
          }
          n361 = Increment(x=w1053) -> (x+1=w1044:i32)
        }
        frame 106 {
          w1071 = "INITIAL_COLUMN "
          n362 = Unbundle By Name(w1065) -> ("lastStatus"=w1066:string)
          n363 = Match Pattern(string=w1066, regular expression=w1071) -> (match substring=w1070:string, after substring=w1068:string)  [unwired: 1 in, 2 out]
          n364 = Equal?(x=w1070, y=w1071) -> (x = y?=w1074:bool)
          n365 = case shown="False" w1074 {
            tunnel: [w1075 w1077] -> w1073
            tunnel: w1072 -> [w1075 w1077]
            tunnel: w1065 -> [w1076 w1083]
            tunnel: [w1076 w1081] -> w1069
            tunnel: w1068 -> [_ w1079]
            frame False {
            }
            frame True {
              n366 = call <vilib>:"Space Constant.vi"() -> ("String"=w1080:string)
              n367 = Match Pattern(string=w1079, regular expression=w1080) -> (before substring=w1078:string)  [unwired: 1 in, 3 out]
              n368 = Fract/Exp String To Number(string=w1078) -> (number=w1082:dbl)  [unwired: 3 in, 1 out]
              n369 = Bundle By Name(cluster=w1083, "InitialColumn"=w1082) -> (w1081:refnum<class "Channel.lvclass">)
            }
          }
          n370 = Increment(x=w1073) -> (x+1=w1064:i32)
        }
        frame 107 {
          w1091 = "FINAL_COLUMN "
          n371 = Unbundle By Name(w1085) -> ("lastStatus"=w1086:string)
          n372 = Match Pattern(string=w1086, regular expression=w1091) -> (match substring=w1090:string, after substring=w1088:string)  [unwired: 1 in, 2 out]
          n373 = Equal?(x=w1090, y=w1091) -> (x = y?=w1094:bool)
          n374 = case shown="True" w1094 {
            tunnel: [w1095 w1097] -> w1093
            tunnel: w1092 -> [w1095 w1097]
            tunnel: w1085 -> [w1096 w1103]
            tunnel: [w1096 w1101] -> w1089
            tunnel: w1088 -> [_ w1099]
            frame False {
            }
            frame True {
              n375 = call <vilib>:"Space Constant.vi"() -> ("String"=w1100:string)
              n376 = Match Pattern(string=w1099, regular expression=w1100) -> (before substring=w1098:string)  [unwired: 1 in, 3 out]
              n377 = Fract/Exp String To Number(string=w1098) -> (number=w1102:dbl)  [unwired: 3 in, 1 out]
              n378 = Bundle By Name(cluster=w1103, "FinalColumn"=w1102) -> (w1101:refnum<class "Channel.lvclass">)
            }
          }
          n379 = Increment(x=w1093) -> (x+1=w1084:i32)
        }
        frame 108 {
          w1111 = "EM_GAIN "
          n380 = Unbundle By Name(w1105) -> ("lastStatus"=w1106:string)
          n381 = Match Pattern(string=w1106, regular expression=w1111) -> (match substring=w1110:string, after substring=w1108:string)  [unwired: 1 in, 2 out]
          n382 = Equal?(x=w1110, y=w1111) -> (x = y?=w1114:bool)
          n383 = case shown="True" w1114 {
            tunnel: [w1115 w1117] -> w1113
            tunnel: w1112 -> [w1115 w1117]
            tunnel: w1105 -> [w1116 w1123]
            tunnel: [w1116 w1121] -> w1109
            tunnel: w1108 -> [_ w1119]
            frame False {
            }
            frame True {
              n384 = call <vilib>:"Space Constant.vi"() -> ("String"=w1120:string)
              n385 = Match Pattern(string=w1119, regular expression=w1120) -> (before substring=w1118:string)  [unwired: 1 in, 3 out]
              n386 = Fract/Exp String To Number(string=w1118) -> (number=w1122:dbl)  [unwired: 3 in, 1 out]
              n387 = Bundle By Name(cluster=w1123, "EmGain"=w1122) -> (w1121:refnum<class "Channel.lvclass">)
            }
          }
          n388 = Increment(x=w1113) -> (x+1=w1104:i32)
        }
        frame 109 {
          w1131 = "COOLER "
          n389 = Unbundle By Name(w1125) -> ("lastStatus"=w1126:string)
          n390 = Match Pattern(string=w1126, regular expression=w1131) -> (match substring=w1130:string, after substring=w1128:string)  [unwired: 1 in, 2 out]
          n391 = Equal?(x=w1130, y=w1131) -> (x = y?=w1134:bool)
          n392 = case shown="True" w1134 {
            tunnel: [w1135 w1137] -> w1133
            tunnel: w1132 -> [w1135 w1137]
            tunnel: w1125 -> [w1136 w1144]
            tunnel: [w1136 w1143] -> w1129
            tunnel: w1128 -> [_ w1141]
            frame False {
            }
            frame True {
              n393 = call <vilib>:"Space Constant.vi"() -> ("String"=w1142:string)
              n394 = Match Pattern(string=w1141, regular expression=w1142) -> (before substring=w1140:string)  [unwired: 1 in, 3 out]
              n395 = Equal?(x=w1140, y="ON") -> (x = y?=w1138:bool)
              n396 = Bundle By Name(cluster=w1144, "Cooler Off"=w1138) -> (w1143:refnum<class "Channel.lvclass">)
            }
          }
          n397 = Increment(x=w1133) -> (x+1=w1124:i32)
        }
        frame 110 {
        }
        frame 200 {
          n398 = Unbundle By Name(w1156) -> ("Interface.lvclass"=w1155:refnum<class "Interface.lvclass">)
          n399 = call "Read Camera Setup.vi"("Interface in"=w1155) -> ("Camera Setup"=w1149:T3)  [unwired: 8 in, 2 out]
          n400 = Unbundle By Name(w1149) -> ("EXPTIME"=w1148:dbl)
          n401 = Number To Fractional String(number=w1148) -> (F-format string=w1150:string)  [unwired: 3 in]
          n402 = Concatenate Strings("SET EXPTIME " ("cmd"), w1150) -> (w1154:string)
          n403 = call-dynamic "Write cmd.vi"("error in (no error)"=w1158, "cmd"=w1154, "Device in"=w1156) -> ("error out"=w1157:errorcluster, "Device out"=w1159:refnum<class "Channel.lvclass">)  [unwired: 7 in]
          n404 = Increment(x=w1152) -> (x+1=w1153:i32)
        }
        frame 201 {
          n405 = call-dynamic "Read resp.vi"("error in (no error)"=w1167, "Device in"=w1168) -> ("error out"=w1161:errorcluster, "resp"=w1166:string, "Device out"=w1162:refnum<class "Channel.lvclass">)  [unwired: 7 in]
          n406 = Equal?(x=w1166, y="DONE") -> (x = y?=w1164:bool)
          n407 = case shown="True" w1164 {
            tunnel: [w1169 w1170] -> w1163
            tunnel: w1160 -> [w1169 w1171]
            frame False {
            }
            frame True {
              n408 = Increment(x=w1171) -> (x+1=w1170:i32)
            }
          }
        }
        frame 202 {
          n409 = call-dynamic "Write cmd.vi"("error in (no error)"=w1177, "cmd"="GET EXPTIME", "Device in"=w1175) -> ("error out"=w1176:errorcluster, "Device out"=w1178:refnum<class "Channel.lvclass">)  [unwired: 7 in]
          n410 = Increment(x=w1173) -> (x+1=w1174:i32)
        }
        frame 203 {
          n411 = call-dynamic "Read resp.vi"("error in (no error)"=w1189, "Device in"=w1190) -> ("error out"=w1187:errorcluster, "resp"=w1182:string, "Device out"=w1185:refnum<class "Channel.lvclass">)  [unwired: 7 in]
          n412 = Fract/Exp String To Number(string=w1182) -> (number=w1179:dbl)  [unwired: 3 in, 1 out]
          n413 = Unbundle By Name(w1185) -> ("Interface.lvclass"=w1184:refnum<class "Interface.lvclass">)
          n414 = call "Read Camera Setup.vi"("Interface in"=w1184) -> ("Camera Setup"=w1183:T3)  [unwired: 8 in, 2 out]
          n415 = Unbundle By Name(w1183) -> ("EXPTIME"=w1180:dbl)
          n416 = Equal?(x=w1180, y=w1179) -> (x = y?=w1181:bool)
          n417 = disable-structure shown="Enabled" {
            disable-tunnel: [w1193 224 ("State")] -> w1188
            disable-tunnel: w1186 -> [w1192 _]
            disable-tunnel: w1181 -> [w1191 _]
            frame Disabled {
              n418 = case shown="True" w1191 {
                tunnel: [w1194 w1195] -> w1193
                tunnel: w1192 -> [w1194 w1196]
                frame False {
                }
                frame True {
                  n419 = Increment(x=w1196) -> (x+1=w1195:i32)
                }
              }
            }
            frame Enabled {
            }
          }
        }
        frame 204 {
          n420 = Unbundle By Name(w1206) -> ("Interface.lvclass"=w1205:refnum<class "Interface.lvclass">)
          n421 = call "Read Camera Setup.vi"("Interface in"=w1205) -> ("Camera Setup"=w1199:T3)  [unwired: 8 in, 2 out]
          n422 = Unbundle By Name(w1199) -> ("#FRAMES"=w1198:u32)
          n423 = Number To Fractional String(number=w1198) -> (F-format string=w1200:string)  [unwired: 3 in]
          n424 = Concatenate Strings("SET #FRAMES " ("cmd"), w1200) -> (w1204:string)
          n425 = call-dynamic "Write cmd.vi"("error in (no error)"=w1208, "cmd"=w1204, "Device in"=w1206) -> ("error out"=w1207:errorcluster, "Device out"=w1209:refnum<class "Channel.lvclass">)  [unwired: 7 in]
          n426 = Increment(x=w1202) -> (x+1=w1203:i32)
        }
        frame 205 {
          n427 = call-dynamic "Read resp.vi"("error in (no error)"=w1217, "Device in"=w1218) -> ("error out"=w1211:errorcluster, "resp"=w1216:string, "Device out"=w1212:refnum<class "Channel.lvclass">)  [unwired: 7 in]
          n428 = Equal?(x=w1216, y="DONE") -> (x = y?=w1214:bool)
          n429 = case shown="True" w1214 {
            tunnel: [w1219 w1220] -> w1213
            tunnel: w1210 -> [w1219 w1221]
            frame False {
            }
            frame True {
              n430 = Increment(x=w1221) -> (x+1=w1220:i32)
            }
          }
        }
        frame 206 {
          n431 = call-dynamic "Write cmd.vi"("error in (no error)"=w1227, "cmd"="GET #FRAMES", "Device in"=w1225) -> ("error out"=w1226:errorcluster, "Device out"=w1228:refnum<class "Channel.lvclass">)  [unwired: 7 in]
          n432 = Increment(x=w1223) -> (x+1=w1224:i32)
        }
        frame 207 {
          n433 = call-dynamic "Read resp.vi"("error in (no error)"=w1240, "Device in"=w1241) -> ("error out"=w1238:errorcluster, "resp"=w1233:string, "Device out"=w1236:refnum<class "Channel.lvclass">)  [unwired: 7 in]
          n434 = Decimal String To Number(string=w1233) -> (number=w1231:i32)  [unwired: 2 in, 1 out]
          n435 = Unbundle By Name(w1236) -> ("Interface.lvclass"=w1235:refnum<class "Interface.lvclass">)
          n436 = call "Read Camera Setup.vi"("Interface in"=w1235) -> ("Camera Setup"=w1234:T3)  [unwired: 8 in, 2 out]
          n437 = To Unsigned Long Integer(number=w1231) -> (unsigned 32bit integer=w1229:u32)
          n438 = Unbundle By Name(w1234) -> ("#FRAMES"=w1230:u32)
          n439 = Equal?(x=w1230, y=w1229) -> (x = y?=w1232:bool)
          n440 = case shown="True" w1232 {
            tunnel: [w1242 w1243] -> w1239
            tunnel: w1237 -> [w1242 w1244]
            frame False {
            }
            frame True {
              n441 = Increment(x=w1244) -> (x+1=w1243:i32)
            }
          }
        }
        frame 208 {
          n442 = Unbundle By Name(w1253) -> ("Interface.lvclass"=w1252:refnum<class "Interface.lvclass">)
          n443 = call "Read Camera Setup.vi"("Interface in"=w1252) -> ("Camera Setup"=w1246:T3)  [unwired: 8 in, 2 out]
          n444 = Unbundle By Name(w1246) -> ("TRIGGER_MODE"=w1245:u8)
          n445 = Number To Fractional String(number=w1245) -> (F-format string=w1247:string)  [unwired: 3 in]
          n446 = Concatenate Strings("SET TRIGGER_MODE " ("cmd"), w1247) -> (w1251:string)
          n447 = call-dynamic "Write cmd.vi"("error in (no error)"=w1255, "cmd"=w1251, "Device in"=w1253) -> ("error out"=w1254:errorcluster, "Device out"=w1256:refnum<class "Channel.lvclass">)  [unwired: 7 in]
          n448 = Increment(x=w1249) -> (x+1=w1250:i32)
        }
        frame 209 {
          n449 = call-dynamic "Read resp.vi"("error in (no error)"=w1264, "Device in"=w1265) -> ("error out"=w1258:errorcluster, "resp"=w1263:string, "Device out"=w1259:refnum<class "Channel.lvclass">)  [unwired: 7 in]
          n450 = Equal?(x=w1263, y="DONE") -> (x = y?=w1261:bool)
          n451 = case shown="True" w1261 {
            tunnel: [w1266 w1267] -> w1260
            tunnel: w1257 -> [w1266 w1268]
            frame False {
            }
            frame True {
              n452 = Increment(x=w1268) -> (x+1=w1267:i32)
            }
          }
        }
        frame 210 {
          n453 = call-dynamic "Write cmd.vi"("error in (no error)"=w1274, "cmd"="GET TRIGGER_MODE", "Device in"=w1272) -> ("error out"=w1273:errorcluster, "Device out"=w1275:refnum<class "Channel.lvclass">)  [unwired: 7 in]
          n454 = Increment(x=w1270) -> (x+1=w1271:i32)
        }
        frame 211 {
          n455 = call-dynamic "Read resp.vi"("error in (no error)"=w1286, "Device in"=w1287) -> ("error out"=w1284:errorcluster, "resp"=w1279:string, "Device out"=w1282:refnum<class "Channel.lvclass">)  [unwired: 7 in]
          n456 = Fract/Exp String To Number(string=w1279) -> (number=w1277:dbl)  [unwired: 3 in, 1 out]
          n457 = Unbundle By Name(w1282) -> ("Interface.lvclass"=w1281:refnum<class "Interface.lvclass">)
          n458 = call "Read Camera Setup.vi"("Interface in"=w1281) -> ("Camera Setup"=w1280:T3)  [unwired: 8 in, 2 out]
          n459 = Unbundle By Name(w1280) -> ("TRIGGER_MODE"=w1276:u8)
          n460 = Equal?(x=w1276, y=w1277) -> (x = y?=w1278:bool)
          n461 = case shown="False" w1278 {
            tunnel: [w1288 w1289] -> w1285
            tunnel: w1283 -> [w1288 w1290]
            frame False {
            }
            frame True {
              n462 = Increment(x=w1290) -> (x+1=w1289:i32)
            }
          }
        }
        frame 212 {
          n463 = Unbundle By Name(w1299) -> ("Interface.lvclass"=w1298:refnum<class "Interface.lvclass">)
          n464 = call "Read Camera Setup.vi"("Interface in"=w1298) -> ("Camera Setup"=w1292:T3)  [unwired: 8 in, 2 out]
          n465 = Unbundle By Name(w1292) -> ("READ_MODE"=w1291:u8)
          n466 = Number To Fractional String(number=w1291) -> (F-format string=w1293:string)  [unwired: 3 in]
          n467 = Concatenate Strings("SET READ_MODE " ("cmd"), w1293) -> (w1297:string)
          n468 = call-dynamic "Write cmd.vi"("error in (no error)"=w1301, "cmd"=w1297, "Device in"=w1299) -> ("error out"=w1300:errorcluster, "Device out"=w1302:refnum<class "Channel.lvclass">)  [unwired: 7 in]
          n469 = Increment(x=w1295) -> (x+1=w1296:i32)
        }
        frame 213 {
          n470 = call-dynamic "Read resp.vi"("error in (no error)"=w1310, "Device in"=w1311) -> ("error out"=w1304:errorcluster, "resp"=w1309:string, "Device out"=w1305:refnum<class "Channel.lvclass">)  [unwired: 7 in]
          n471 = Equal?(x=w1309, y="DONE") -> (x = y?=w1307:bool)
          n472 = case shown="True" w1307 {
            tunnel: [w1312 w1313] -> w1306
            tunnel: w1303 -> [w1312 w1314]
            frame False {
            }
            frame True {
              n473 = Increment(x=w1314) -> (x+1=w1313:i32)
            }
          }
        }
        frame 214 {
          n474 = call-dynamic "Write cmd.vi"("error in (no error)"=w1320, "cmd"="GET READ_MODE", "Device in"=w1318) -> ("error out"=w1319:errorcluster, "Device out"=w1321:refnum<class "Channel.lvclass">)  [unwired: 7 in]
          n475 = Increment(x=w1316) -> (x+1=w1317:i32)
        }
        frame 215 {
          n476 = call-dynamic "Read resp.vi"("error in (no error)"=w1332, "Device in"=w1333) -> ("error out"=w1330:errorcluster, "resp"=w1325:string, "Device out"=w1328:refnum<class "Channel.lvclass">)  [unwired: 7 in]
          n477 = Fract/Exp String To Number(string=w1325) -> (number=w1323:dbl)  [unwired: 3 in, 1 out]
          n478 = Unbundle By Name(w1328) -> ("Interface.lvclass"=w1327:refnum<class "Interface.lvclass">)
          n479 = call "Read Camera Setup.vi"("Interface in"=w1327) -> ("Camera Setup"=w1326:T3)  [unwired: 8 in, 2 out]
          n480 = Unbundle By Name(w1326) -> ("READ_MODE"=w1322:u8)
          n481 = Equal?(x=w1322, y=w1323) -> (x = y?=w1324:bool)
          n482 = case shown="True" w1324 {
            tunnel: [w1334 w1335] -> w1331
            tunnel: w1329 -> [w1334 w1336]
            frame False {
            }
            frame True {
              n483 = Increment(x=w1336) -> (x+1=w1335:i32)
            }
          }
        }
        frame 216 {
          n484 = Unbundle By Name(w1345) -> ("Interface.lvclass"=w1344:refnum<class "Interface.lvclass">)
          n485 = call "Read Camera Setup.vi"("Interface in"=w1344) -> ("Camera Setup"=w1338:T3)  [unwired: 8 in, 2 out]
          n486 = Unbundle By Name(w1338) -> ("READOUT_RATE"=w1337:u8)
          n487 = Number To Fractional String(number=w1337) -> (F-format string=w1339:string)  [unwired: 3 in]
          n488 = Concatenate Strings("SET READOUT_RATE " ("cmd"), w1339) -> (w1343:string)
          n489 = call-dynamic "Write cmd.vi"("error in (no error)"=w1347, "cmd"=w1343, "Device in"=w1345) -> ("error out"=w1346:errorcluster, "Device out"=w1348:refnum<class "Channel.lvclass">)  [unwired: 7 in]
          n490 = Increment(x=w1341) -> (x+1=w1342:i32)
        }
        frame 217 {
          n491 = call-dynamic "Read resp.vi"("error in (no error)"=w1356, "Device in"=w1357) -> ("error out"=w1350:errorcluster, "resp"=w1355:string, "Device out"=w1351:refnum<class "Channel.lvclass">)  [unwired: 7 in]
          n492 = Equal?(x=w1355, y="DONE") -> (x = y?=w1353:bool)
          n493 = case shown="True" w1353 {
            tunnel: [w1358 w1359] -> w1352
            tunnel: w1349 -> [w1358 w1360]
            frame False {
            }
            frame True {
              n494 = Increment(x=w1360) -> (x+1=w1359:i32)
            }
          }
        }
        frame 218 {
          n495 = call-dynamic "Write cmd.vi"("error in (no error)"=w1366, "cmd"="GET READOUT_RATE", "Device in"=w1364) -> ("error out"=w1365:errorcluster, "Device out"=w1367:refnum<class "Channel.lvclass">)  [unwired: 7 in]
          n496 = Increment(x=w1362) -> (x+1=w1363:i32)
        }
        frame 219 {
          n497 = call-dynamic "Read resp.vi"("error in (no error)"=w1378, "Device in"=w1379) -> ("error out"=w1376:errorcluster, "resp"=w1371:string, "Device out"=w1374:refnum<class "Channel.lvclass">)  [unwired: 7 in]
          n498 = Fract/Exp String To Number(string=w1371) -> (number=w1369:dbl)  [unwired: 3 in, 1 out]
          n499 = Unbundle By Name(w1374) -> ("Interface.lvclass"=w1373:refnum<class "Interface.lvclass">)
          n500 = call "Read Camera Setup.vi"("Interface in"=w1373) -> ("Camera Setup"=w1372:T3)  [unwired: 8 in, 2 out]
          n501 = Unbundle By Name(w1372) -> ("READOUT_RATE"=w1368:u8)
          n502 = Equal?(x=w1368, y=w1369) -> (x = y?=w1370:bool)
          n503 = case shown="True" w1370 {
            tunnel: [w1380 w1381] -> w1377
            tunnel: w1375 -> [w1380 w1382]
            frame False {
            }
            frame True {
              n504 = Increment(x=w1382) -> (x+1=w1381:i32)
            }
          }
        }
        frame 220 {
          n505 = Unbundle By Name(w1391) -> ("Interface.lvclass"=w1390:refnum<class "Interface.lvclass">)
          n506 = call "Read Camera Setup.vi"("Interface in"=w1390) -> ("Camera Setup"=w1384:T3)  [unwired: 8 in, 2 out]
          n507 = Unbundle By Name(w1384) -> ("VERTICAL_SHIFT_SPEED"=w1383:u8)
          n508 = Number To Fractional String(number=w1383) -> (F-format string=w1385:string)  [unwired: 3 in]
          n509 = Concatenate Strings("SET VERTICAL_SHIFT_SPEED " ("cmd"), w1385) -> (w1389:string)
          n510 = call-dynamic "Write cmd.vi"("error in (no error)"=w1393, "cmd"=w1389, "Device in"=w1391) -> ("error out"=w1392:errorcluster, "Device out"=w1394:refnum<class "Channel.lvclass">)  [unwired: 7 in]
          n511 = Increment(x=w1387) -> (x+1=w1388:i32)
        }
        frame 221 {
          n512 = call-dynamic "Read resp.vi"("error in (no error)"=w1402, "Device in"=w1403) -> ("error out"=w1396:errorcluster, "resp"=w1401:string, "Device out"=w1397:refnum<class "Channel.lvclass">)  [unwired: 7 in]
          n513 = Equal?(x=w1401, y="DONE") -> (x = y?=w1399:bool)
          n514 = case shown="True" w1399 {
            tunnel: [w1404 w1405] -> w1398
            tunnel: w1395 -> [w1404 w1406]
            frame False {
            }
            frame True {
              n515 = Increment(x=w1406) -> (x+1=w1405:i32)
            }
          }
        }
        frame 222 {
          n516 = call-dynamic "Write cmd.vi"("error in (no error)"=w1412, "cmd"="GET VERTICAL_SHIFT_SPEED", "Device in"=w1410) -> ("error out"=w1411:errorcluster, "Device out"=w1413:refnum<class "Channel.lvclass">)  [unwired: 7 in]
          n517 = Increment(x=w1408) -> (x+1=w1409:i32)
        }
        frame 223 {
          n518 = call-dynamic "Read resp.vi"("error in (no error)"=w1424, "Device in"=w1425) -> ("error out"=w1422:errorcluster, "resp"=w1417:string, "Device out"=w1420:refnum<class "Channel.lvclass">)  [unwired: 7 in]
          n519 = Fract/Exp String To Number(string=w1417) -> (number=w1415:dbl)  [unwired: 3 in, 1 out]
          n520 = Unbundle By Name(w1420) -> ("Interface.lvclass"=w1419:refnum<class "Interface.lvclass">)
          n521 = call "Read Camera Setup.vi"("Interface in"=w1419) -> ("Camera Setup"=w1418:T3)  [unwired: 8 in, 2 out]
          n522 = Unbundle By Name(w1418) -> ("VERTICAL_SHIFT_SPEED"=w1414:u8)
          n523 = Equal?(x=w1414, y=w1415) -> (x = y?=w1416:bool)
          n524 = case shown="True" w1416 {
            tunnel: [w1426 w1427] -> w1423
            tunnel: w1421 -> [w1426 w1428]
            frame False {
            }
            frame True {
              n525 = Increment(x=w1428) -> (x+1=w1427:i32)
            }
          }
        }
        frame 224 {
          n526 = Unbundle By Name(w1437) -> ("Interface.lvclass"=w1436:refnum<class "Interface.lvclass">)
          n527 = call "Read Camera Setup.vi"("Interface in"=w1436) -> ("Camera Setup"=w1430:T3)  [unwired: 8 in, 2 out]
          n528 = Unbundle By Name(w1430) -> ("PREAMP"=w1429:u8)
          n529 = Number To Fractional String(number=w1429) -> (F-format string=w1431:string)  [unwired: 3 in]
          n530 = Concatenate Strings("SET PREAMP " ("cmd"), w1431) -> (w1435:string)
          n531 = call-dynamic "Write cmd.vi"("error in (no error)"=w1439, "cmd"=w1435, "Device in"=w1437) -> ("error out"=w1438:errorcluster, "Device out"=w1440:refnum<class "Channel.lvclass">)  [unwired: 7 in]
          n532 = Increment(x=w1433) -> (x+1=w1434:i32)
        }
        frame 225 {
          n533 = call-dynamic "Read resp.vi"("error in (no error)"=w1448, "Device in"=w1449) -> ("error out"=w1442:errorcluster, "resp"=w1447:string, "Device out"=w1443:refnum<class "Channel.lvclass">)  [unwired: 7 in]
          n534 = Equal?(x=w1447, y="DONE") -> (x = y?=w1445:bool)
          n535 = case shown="True" w1445 {
            tunnel: [w1450 w1451] -> w1444
            tunnel: w1441 -> [w1450 w1452]
            frame False {
            }
            frame True {
              n536 = Increment(x=w1452) -> (x+1=w1451:i32)
            }
          }
        }
        frame 226 {
          n537 = call-dynamic "Write cmd.vi"("error in (no error)"=w1458, "cmd"="GET PREAMP", "Device in"=w1456) -> ("error out"=w1457:errorcluster, "Device out"=w1459:refnum<class "Channel.lvclass">)  [unwired: 7 in]
          n538 = Increment(x=w1454) -> (x+1=w1455:i32)
        }
        frame 227 {
          n539 = call-dynamic "Read resp.vi"("error in (no error)"=w1470, "Device in"=w1471) -> ("error out"=w1468:errorcluster, "resp"=w1463:string, "Device out"=w1466:refnum<class "Channel.lvclass">)  [unwired: 7 in]
          n540 = Fract/Exp String To Number(string=w1463) -> (number=w1461:dbl)  [unwired: 3 in, 1 out]
          n541 = Unbundle By Name(w1466) -> ("Interface.lvclass"=w1465:refnum<class "Interface.lvclass">)
          n542 = call "Read Camera Setup.vi"("Interface in"=w1465) -> ("Camera Setup"=w1464:T3)  [unwired: 8 in, 2 out]
          n543 = Unbundle By Name(w1464) -> ("PREAMP"=w1460:u8)
          n544 = Equal?(x=w1460, y=w1461) -> (x = y?=w1462:bool)
          n545 = case shown="True" w1462 {
            tunnel: [w1472 w1473] -> w1469
            tunnel: w1467 -> [w1472 w1474]
            frame False {
            }
            frame True {
              n546 = Increment(x=w1474) -> (x+1=w1473:i32)
            }
          }
        }
        frame 228 {
          n547 = Unbundle By Name(w1483) -> ("Interface.lvclass"=w1482:refnum<class "Interface.lvclass">)
          n548 = call "Read Camera Setup.vi"("Interface in"=w1482) -> ("Camera Setup"=w1476:T3)  [unwired: 8 in, 2 out]
          n549 = Unbundle By Name(w1476) -> ("EM_MODE"=w1475:u8)
          n550 = Number To Fractional String(number=w1475) -> (F-format string=w1477:string)  [unwired: 3 in]
          n551 = Concatenate Strings("SET EM_MODE " ("cmd"), w1477) -> (w1481:string)
          n552 = call-dynamic "Write cmd.vi"("error in (no error)"=w1485, "cmd"=w1481, "Device in"=w1483) -> ("error out"=w1484:errorcluster, "Device out"=w1486:refnum<class "Channel.lvclass">)  [unwired: 7 in]
          n553 = Increment(x=w1479) -> (x+1=w1480:i32)
        }
        frame 229 {
          n554 = call-dynamic "Read resp.vi"("error in (no error)"=w1494, "Device in"=w1495) -> ("error out"=w1488:errorcluster, "resp"=w1493:string, "Device out"=w1489:refnum<class "Channel.lvclass">)  [unwired: 7 in]
          n555 = Equal?(x=w1493, y="DONE") -> (x = y?=w1491:bool)
          n556 = case shown="True" w1491 {
            tunnel: [w1496 w1497] -> w1490
            tunnel: w1487 -> [w1496 w1498]
            frame False {
            }
            frame True {
              n557 = Increment(x=w1498) -> (x+1=w1497:i32)
            }
          }
        }
        frame 230 {
          n558 = call-dynamic "Write cmd.vi"("error in (no error)"=w1504, "cmd"="GET EM_MODE", "Device in"=w1502) -> ("error out"=w1503:errorcluster, "Device out"=w1505:refnum<class "Channel.lvclass">)  [unwired: 7 in]
          n559 = Increment(x=w1500) -> (x+1=w1501:i32)
        }
        frame 231 {
          n560 = call-dynamic "Read resp.vi"("error in (no error)"=w1516, "Device in"=w1517) -> ("error out"=w1514:errorcluster, "resp"=w1509:string, "Device out"=w1512:refnum<class "Channel.lvclass">)  [unwired: 7 in]
          n561 = Fract/Exp String To Number(string=w1509) -> (number=w1507:dbl)  [unwired: 3 in, 1 out]
          n562 = Unbundle By Name(w1512) -> ("Interface.lvclass"=w1511:refnum<class "Interface.lvclass">)
          n563 = call "Read Camera Setup.vi"("Interface in"=w1511) -> ("Camera Setup"=w1510:T3)  [unwired: 8 in, 2 out]
          n564 = Unbundle By Name(w1510) -> ("EM_MODE"=w1506:u8)
          n565 = Equal?(x=w1506, y=w1507) -> (x = y?=w1508:bool)
          n566 = case shown="True" w1508 {
            tunnel: [w1518 w1519] -> w1515
            tunnel: w1513 -> [w1518 w1520]
            frame False {
            }
            frame True {
              n567 = Increment(x=w1520) -> (x+1=w1519:i32)
            }
          }
        }
        frame 232 {
          n568 = Unbundle By Name(w1529) -> ("Interface.lvclass"=w1528:refnum<class "Interface.lvclass">)
          n569 = call "Read Camera Setup.vi"("Interface in"=w1528) -> ("Camera Setup"=w1522:T3)  [unwired: 8 in, 2 out]
          n570 = Unbundle By Name(w1522) -> ("EM_GAIN"=w1521:u16)
          n571 = Number To Fractional String(number=w1521) -> (F-format string=w1523:string)  [unwired: 3 in]
          n572 = Concatenate Strings("SET EM_GAIN " ("cmd"), w1523) -> (w1527:string)
          n573 = call-dynamic "Write cmd.vi"("error in (no error)"=w1531, "cmd"=w1527, "Device in"=w1529) -> ("error out"=w1530:errorcluster, "Device out"=w1532:refnum<class "Channel.lvclass">)  [unwired: 7 in]
          n574 = Increment(x=w1525) -> (x+1=w1526:i32)
        }
        frame 233 {
          n575 = call-dynamic "Read resp.vi"("error in (no error)"=w1540, "Device in"=w1541) -> ("error out"=w1534:errorcluster, "resp"=w1539:string, "Device out"=w1535:refnum<class "Channel.lvclass">)  [unwired: 7 in]
          n576 = Equal?(x=w1539, y="DONE") -> (x = y?=w1537:bool)
          n577 = case shown="True" w1537 {
            tunnel: [w1542 w1543] -> w1536
            tunnel: w1533 -> [w1542 w1544]
            frame False {
            }
            frame True {
              n578 = Increment(x=w1544) -> (x+1=w1543:i32)
            }
          }
        }
        frame 234 {
          n579 = call-dynamic "Write cmd.vi"("error in (no error)"=w1550, "cmd"="GET EM_GAIN", "Device in"=w1548) -> ("error out"=w1549:errorcluster, "Device out"=w1551:refnum<class "Channel.lvclass">)  [unwired: 7 in]
          n580 = Increment(x=w1546) -> (x+1=w1547:i32)
        }
        frame 235 {
          n581 = call-dynamic "Read resp.vi"("error in (no error)"=w1562, "Device in"=w1563) -> ("error out"=w1560:errorcluster, "resp"=w1555:string, "Device out"=w1558:refnum<class "Channel.lvclass">)  [unwired: 7 in]
          n582 = Fract/Exp String To Number(string=w1555) -> (number=w1553:dbl)  [unwired: 3 in, 1 out]
          n583 = Unbundle By Name(w1558) -> ("Interface.lvclass"=w1557:refnum<class "Interface.lvclass">)
          n584 = call "Read Camera Setup.vi"("Interface in"=w1557) -> ("Camera Setup"=w1556:T3)  [unwired: 8 in, 2 out]
          n585 = Unbundle By Name(w1556) -> ("EM_GAIN"=w1552:u16)
          n586 = Equal?(x=w1552, y=w1553) -> (x = y?=w1554:bool)
          n587 = disable-structure shown="Enabled" {
            disable-tunnel: [w1566 264 ("State")] -> w1561
            disable-tunnel: w1559 -> [w1565 _]
            disable-tunnel: w1554 -> [w1564 _]
            frame Disabled {
              n588 = case shown="True" w1564 {
                tunnel: [w1567 w1568] -> w1566
                tunnel: w1565 -> [w1567 w1569]
                frame False {
                }
                frame True {
                  n589 = Increment(x=w1569) -> (x+1=w1568:i32)
                }
              }
            }
            frame Enabled {
            }
          }
        }
        frame 236 {
          n590 = Unbundle By Name(w1579) -> ("Interface.lvclass"=w1578:refnum<class "Interface.lvclass">)
          n591 = call "Read Camera Setup.vi"("Interface in"=w1578) -> ("Camera Setup"=w1572:T3)  [unwired: 8 in, 2 out]
          n592 = Unbundle By Name(w1572) -> ("ACQUISITION_MODE"=w1571:u8)
          n593 = Number To Fractional String(number=w1571) -> (F-format string=w1573:string)  [unwired: 3 in]
          n594 = Concatenate Strings("SET ACQUISITION_MODE " ("cmd"), w1573) -> (w1577:string)
          n595 = call-dynamic "Write cmd.vi"("error in (no error)"=w1581, "cmd"=w1577, "Device in"=w1579) -> ("error out"=w1580:errorcluster, "Device out"=w1582:refnum<class "Channel.lvclass">)  [unwired: 7 in]
          n596 = Increment(x=w1575) -> (x+1=w1576:i32)
        }
        frame 237 {
          n597 = call-dynamic "Read resp.vi"("error in (no error)"=w1590, "Device in"=w1591) -> ("error out"=w1584:errorcluster, "resp"=w1589:string, "Device out"=w1585:refnum<class "Channel.lvclass">)  [unwired: 7 in]
          n598 = Equal?(x=w1589, y="DONE") -> (x = y?=w1587:bool)
          n599 = case shown="True" w1587 {
            tunnel: [w1592 w1593] -> w1586
            tunnel: w1583 -> [w1592 w1594]
            frame False {
            }
            frame True {
              n600 = Increment(x=w1594) -> (x+1=w1593:i32)
            }
          }
        }
        frame 238 {
          n601 = call-dynamic "Write cmd.vi"("error in (no error)"=w1600, "cmd"="GET ACQUISITION_MODE", "Device in"=w1598) -> ("error out"=w1599:errorcluster, "Device out"=w1601:refnum<class "Channel.lvclass">)  [unwired: 7 in]
          n602 = Increment(x=w1596) -> (x+1=w1597:i32)
        }
        frame 239 {
          n603 = call-dynamic "Read resp.vi"("error in (no error)"=w1612, "Device in"=w1613) -> ("error out"=w1610:errorcluster, "resp"=w1605:string, "Device out"=w1608:refnum<class "Channel.lvclass">)  [unwired: 7 in]
          n604 = Fract/Exp String To Number(string=w1605) -> (number=w1603:dbl)  [unwired: 3 in, 1 out]
          n605 = Unbundle By Name(w1608) -> ("Interface.lvclass"=w1607:refnum<class "Interface.lvclass">)
          n606 = call "Read Camera Setup.vi"("Interface in"=w1607) -> ("Camera Setup"=w1606:T3)  [unwired: 8 in, 2 out]
          n607 = Unbundle By Name(w1606) -> ("ACQUISITION_MODE"=w1602:u8)
          n608 = Equal?(x=w1602, y=w1603) -> (x = y?=w1604:bool)
          n609 = case shown="True" w1604 {
            tunnel: [w1614 w1615] -> w1611
            tunnel: w1609 -> [w1614 w1616]
            frame False {
            }
            frame True {
              n610 = Increment(x=w1616) -> (x+1=w1615:i32)
            }
          }
        }
        frame 240 {
          n611 = Unbundle By Name(w1625) -> ("Interface.lvclass"=w1624:refnum<class "Interface.lvclass">)
          n612 = call "Read Camera Setup.vi"("Interface in"=w1624) -> ("Camera Setup"=w1618:T3)  [unwired: 8 in, 2 out]
          n613 = Unbundle By Name(w1618) -> ("SHUTTER_MODE"=w1617:u8)
          n614 = Number To Fractional String(number=w1617) -> (F-format string=w1619:string)  [unwired: 3 in]
          n615 = Concatenate Strings("SET SHUTTER_MODE " ("cmd"), w1619) -> (w1623:string)
          n616 = call-dynamic "Write cmd.vi"("error in (no error)"=w1627, "cmd"=w1623, "Device in"=w1625) -> ("error out"=w1626:errorcluster, "Device out"=w1628:refnum<class "Channel.lvclass">)  [unwired: 7 in]
          n617 = Increment(x=w1621) -> (x+1=w1622:i32)
        }
        frame 241 {
          n618 = call-dynamic "Read resp.vi"("error in (no error)"=w1636, "Device in"=w1637) -> ("error out"=w1630:errorcluster, "resp"=w1635:string, "Device out"=w1631:refnum<class "Channel.lvclass">)  [unwired: 7 in]
          n619 = Equal?(x=w1635, y="DONE") -> (x = y?=w1633:bool)
          n620 = case shown="True" w1633 {
            tunnel: [w1638 w1639] -> w1632
            tunnel: w1629 -> [w1638 w1640]
            frame False {
            }
            frame True {
              n621 = Increment(x=w1640) -> (x+1=w1639:i32)
            }
          }
        }
        frame 242 {
          n622 = call-dynamic "Write cmd.vi"("error in (no error)"=w1646, "cmd"="GET SHUTTER_MODE", "Device in"=w1644) -> ("error out"=w1645:errorcluster, "Device out"=w1647:refnum<class "Channel.lvclass">)  [unwired: 7 in]
          n623 = Increment(x=w1642) -> (x+1=w1643:i32)
        }
        frame 243 {
          n624 = call-dynamic "Read resp.vi"("error in (no error)"=w1658, "Device in"=w1659) -> ("error out"=w1656:errorcluster, "resp"=w1651:string, "Device out"=w1654:refnum<class "Channel.lvclass">)  [unwired: 7 in]
          n625 = Fract/Exp String To Number(string=w1651) -> (number=w1649:dbl)  [unwired: 3 in, 1 out]
          n626 = Unbundle By Name(w1654) -> ("Interface.lvclass"=w1653:refnum<class "Interface.lvclass">)
          n627 = call "Read Camera Setup.vi"("Interface in"=w1653) -> ("Camera Setup"=w1652:T3)  [unwired: 8 in, 2 out]
          n628 = Unbundle By Name(w1652) -> ("SHUTTER_MODE"=w1648:u8)
          n629 = Equal?(x=w1648, y=w1649) -> (x = y?=w1650:bool)
          n630 = case shown="True" w1650 {
            tunnel: [w1660 w1661] -> w1657
            tunnel: w1655 -> [w1660 w1662]
            frame False {
            }
            frame True {
              n631 = Increment(x=w1662) -> (x+1=w1661:i32)
            }
          }
        }
        frame 244 {
          n632 = Unbundle By Name(w1671) -> ("Interface.lvclass"=w1670:refnum<class "Interface.lvclass">)
          n633 = call "Read Camera Setup.vi"("Interface in"=w1670) -> ("Camera Setup"=w1664:T3)  [unwired: 8 in, 2 out]
          n634 = Unbundle By Name(w1664) -> ("SHUTTER_TTL"=w1663:u8)
          n635 = Number To Fractional String(number=w1663) -> (F-format string=w1665:string)  [unwired: 3 in]
          n636 = Concatenate Strings("SET SHUTTER_TTL " ("cmd"), w1665) -> (w1669:string)
          n637 = call-dynamic "Write cmd.vi"("error in (no error)"=w1673, "cmd"=w1669, "Device in"=w1671) -> ("error out"=w1672:errorcluster, "Device out"=w1674:refnum<class "Channel.lvclass">)  [unwired: 7 in]
          n638 = Increment(x=w1667) -> (x+1=w1668:i32)
        }
        frame 245 {
          n639 = call-dynamic "Read resp.vi"("error in (no error)"=w1682, "Device in"=w1683) -> ("error out"=w1676:errorcluster, "resp"=w1681:string, "Device out"=w1677:refnum<class "Channel.lvclass">)  [unwired: 7 in]
          n640 = Equal?(x=w1681, y="DONE") -> (x = y?=w1679:bool)
          n641 = case shown="True" w1679 {
            tunnel: [w1684 w1685] -> w1678
            tunnel: w1675 -> [w1684 w1686]
            frame False {
            }
            frame True {
              n642 = Increment(x=w1686) -> (x+1=w1685:i32)
            }
          }
        }
        frame 246 {
          n643 = call-dynamic "Write cmd.vi"("error in (no error)"=w1692, "cmd"="GET SHUTTER_TTL", "Device in"=w1690) -> ("error out"=w1691:errorcluster, "Device out"=w1693:refnum<class "Channel.lvclass">)  [unwired: 7 in]
          n644 = Increment(x=w1688) -> (x+1=w1689:i32)
        }
        frame 247 {
          n645 = call-dynamic "Read resp.vi"("error in (no error)"=w1704, "Device in"=w1705) -> ("error out"=w1702:errorcluster, "resp"=w1697:string, "Device out"=w1700:refnum<class "Channel.lvclass">)  [unwired: 7 in]
          n646 = Fract/Exp String To Number(string=w1697) -> (number=w1695:dbl)  [unwired: 3 in, 1 out]
          n647 = Unbundle By Name(w1700) -> ("Interface.lvclass"=w1699:refnum<class "Interface.lvclass">)
          n648 = call "Read Camera Setup.vi"("Interface in"=w1699) -> ("Camera Setup"=w1698:T3)  [unwired: 8 in, 2 out]
          n649 = Unbundle By Name(w1698) -> ("SHUTTER_TTL"=w1694:u8)
          n650 = Equal?(x=w1694, y=w1695) -> (x = y?=w1696:bool)
          n651 = case shown="True" w1696 {
            tunnel: [w1706 w1707] -> w1703
            tunnel: w1701 -> [w1706 w1708]
            frame False {
            }
            frame True {
              n652 = Increment(x=w1708) -> (x+1=w1707:i32)
            }
          }
        }
        frame 248 {
          n653 = Unbundle By Name(w1717) -> ("Interface.lvclass"=w1716:refnum<class "Interface.lvclass">)
          n654 = call "Read Camera Setup.vi"("Interface in"=w1716) -> ("Camera Setup"=w1710:T3)  [unwired: 8 in, 2 out]
          n655 = Unbundle By Name(w1710) -> ("SHUTTER_OPENNING_TIME"=w1709:u16)
          n656 = Number To Fractional String(number=w1709) -> (F-format string=w1711:string)  [unwired: 3 in]
          n657 = Concatenate Strings("SET SHUTTER_OPENNING_TIME " ("cmd"), w1711) -> (w1715:string)
          n658 = call-dynamic "Write cmd.vi"("error in (no error)"=w1719, "cmd"=w1715, "Device in"=w1717) -> ("error out"=w1718:errorcluster, "Device out"=w1720:refnum<class "Channel.lvclass">)  [unwired: 7 in]
          n659 = Increment(x=w1713) -> (x+1=w1714:i32)
        }
        frame 249 {
          n660 = call-dynamic "Read resp.vi"("error in (no error)"=w1728, "Device in"=w1729) -> ("error out"=w1722:errorcluster, "resp"=w1727:string, "Device out"=w1723:refnum<class "Channel.lvclass">)  [unwired: 7 in]
          n661 = Equal?(x=w1727, y="DONE") -> (x = y?=w1725:bool)
          n662 = case shown="True" w1725 {
            tunnel: [w1730 w1731] -> w1724
            tunnel: w1721 -> [w1730 w1732]
            frame False {
            }
            frame True {
              n663 = Increment(x=w1732) -> (x+1=w1731:i32)
            }
          }
        }
        frame 250 {
          n664 = call-dynamic "Write cmd.vi"("error in (no error)"=w1738, "cmd"="GET SHUTTER_OPENNING_TIME", "Device in"=w1736) -> ("error out"=w1737:errorcluster, "Device out"=w1739:refnum<class "Channel.lvclass">)  [unwired: 7 in]
          n665 = Increment(x=w1734) -> (x+1=w1735:i32)
        }
        frame 251 {
          n666 = call-dynamic "Read resp.vi"("error in (no error)"=w1750, "Device in"=w1751) -> ("error out"=w1748:errorcluster, "resp"=w1743:string, "Device out"=w1746:refnum<class "Channel.lvclass">)  [unwired: 7 in]
          n667 = Fract/Exp String To Number(string=w1743) -> (number=w1741:dbl)  [unwired: 3 in, 1 out]
          n668 = Unbundle By Name(w1746) -> ("Interface.lvclass"=w1745:refnum<class "Interface.lvclass">)
          n669 = call "Read Camera Setup.vi"("Interface in"=w1745) -> ("Camera Setup"=w1744:T3)  [unwired: 8 in, 2 out]
          n670 = Unbundle By Name(w1744) -> ("SHUTTER_OPENNING_TIME"=w1740:u16)
          n671 = Equal?(x=w1740, y=w1741) -> (x = y?=w1742:bool)
          n672 = case shown="True" w1742 {
            tunnel: [w1752 w1753] -> w1749
            tunnel: w1747 -> [w1752 w1754]
            frame False {
            }
            frame True {
              n673 = Increment(x=w1754) -> (x+1=w1753:i32)
            }
          }
        }
        frame 252 {
          n674 = Unbundle By Name(w1763) -> ("Interface.lvclass"=w1762:refnum<class "Interface.lvclass">)
          n675 = call "Read Camera Setup.vi"("Interface in"=w1762) -> ("Camera Setup"=w1756:T3)  [unwired: 8 in, 2 out]
          n676 = Unbundle By Name(w1756) -> ("SHUTTER_CLOSING_TIME"=w1755:u16)
          n677 = Number To Fractional String(number=w1755) -> (F-format string=w1757:string)  [unwired: 3 in]
          n678 = Concatenate Strings("SET SHUTTER_CLOSING_TIME " ("cmd"), w1757) -> (w1761:string)
          n679 = call-dynamic "Write cmd.vi"("error in (no error)"=w1765, "cmd"=w1761, "Device in"=w1763) -> ("error out"=w1764:errorcluster, "Device out"=w1766:refnum<class "Channel.lvclass">)  [unwired: 7 in]
          n680 = Increment(x=w1759) -> (x+1=w1760:i32)
        }
        frame 253 {
          n681 = call-dynamic "Read resp.vi"("error in (no error)"=w1774, "Device in"=w1775) -> ("error out"=w1768:errorcluster, "resp"=w1773:string, "Device out"=w1769:refnum<class "Channel.lvclass">)  [unwired: 7 in]
          n682 = Equal?(x=w1773, y="DONE") -> (x = y?=w1771:bool)
          n683 = case shown="True" w1771 {
            tunnel: [w1776 w1777] -> w1770
            tunnel: w1767 -> [w1776 w1778]
            frame False {
            }
            frame True {
              n684 = Increment(x=w1778) -> (x+1=w1777:i32)
            }
          }
        }
        frame 254 {
          n685 = call-dynamic "Write cmd.vi"("error in (no error)"=w1784, "cmd"="GET SHUTTER_CLOSING_TIME", "Device in"=w1782) -> ("error out"=w1783:errorcluster, "Device out"=w1785:refnum<class "Channel.lvclass">)  [unwired: 7 in]
          n686 = Increment(x=w1780) -> (x+1=w1781:i32)
        }
        frame 255 {
          n687 = call-dynamic "Read resp.vi"("error in (no error)"=w1796, "Device in"=w1797) -> ("error out"=w1794:errorcluster, "resp"=w1789:string, "Device out"=w1792:refnum<class "Channel.lvclass">)  [unwired: 7 in]
          n688 = Fract/Exp String To Number(string=w1789) -> (number=w1787:dbl)  [unwired: 3 in, 1 out]
          n689 = Unbundle By Name(w1792) -> ("Interface.lvclass"=w1791:refnum<class "Interface.lvclass">)
          n690 = call "Read Camera Setup.vi"("Interface in"=w1791) -> ("Camera Setup"=w1790:T3)  [unwired: 8 in, 2 out]
          n691 = Unbundle By Name(w1790) -> ("SHUTTER_CLOSING_TIME"=w1786:u16)
          n692 = Equal?(x=w1786, y=w1787) -> (x = y?=w1788:bool)
          n693 = case shown="True" w1788 {
            tunnel: [w1798 w1799] -> w1795
            tunnel: w1793 -> [w1798 w1800]
            frame False {
            }
            frame True {
              n694 = Increment(x=w1800) -> (x+1=w1799:i32)
            }
          }
        }
        frame 256 {
          n695 = Unbundle By Name(w1809) -> ("Interface.lvclass"=w1808:refnum<class "Interface.lvclass">)
          n696 = call "Read Camera Setup.vi"("Interface in"=w1808) -> ("Camera Setup"=w1802:T3)  [unwired: 8 in, 2 out]
          n697 = Unbundle By Name(w1802) -> ("HBIN"=w1801:u16)
          n698 = Number To Fractional String(number=w1801) -> (F-format string=w1803:string)  [unwired: 3 in]
          n699 = Concatenate Strings("SET HBIN " ("cmd"), w1803) -> (w1807:string)
          n700 = call-dynamic "Write cmd.vi"("error in (no error)"=w1811, "cmd"=w1807, "Device in"=w1809) -> ("error out"=w1810:errorcluster, "Device out"=w1812:refnum<class "Channel.lvclass">)  [unwired: 7 in]
          n701 = Increment(x=w1805) -> (x+1=w1806:i32)
        }
        frame 257 {
          n702 = call-dynamic "Read resp.vi"("error in (no error)"=w1820, "Device in"=w1821) -> ("error out"=w1814:errorcluster, "resp"=w1819:string, "Device out"=w1815:refnum<class "Channel.lvclass">)  [unwired: 7 in]
          n703 = Equal?(x=w1819, y="DONE") -> (x = y?=w1817:bool)
          n704 = case shown="True" w1817 {
            tunnel: [w1822 w1823] -> w1816
            tunnel: w1813 -> [w1822 w1824]
            frame False {
            }
            frame True {
              n705 = Increment(x=w1824) -> (x+1=w1823:i32)
            }
          }
        }
        frame 258 {
          n706 = call-dynamic "Write cmd.vi"("error in (no error)"=w1830, "cmd"="GET HBIN", "Device in"=w1828) -> ("error out"=w1829:errorcluster, "Device out"=w1831:refnum<class "Channel.lvclass">)  [unwired: 7 in]
          n707 = Increment(x=w1826) -> (x+1=w1827:i32)
        }
        frame 259 {
          n708 = call-dynamic "Read resp.vi"("error in (no error)"=w1842, "Device in"=w1843) -> ("error out"=w1840:errorcluster, "resp"=w1835:string, "Device out"=w1838:refnum<class "Channel.lvclass">)  [unwired: 7 in]
          n709 = Fract/Exp String To Number(string=w1835) -> (number=w1833:dbl)  [unwired: 3 in, 1 out]
          n710 = Unbundle By Name(w1838) -> ("Interface.lvclass"=w1837:refnum<class "Interface.lvclass">)
          n711 = call "Read Camera Setup.vi"("Interface in"=w1837) -> ("Camera Setup"=w1836:T3)  [unwired: 8 in, 2 out]
          n712 = Unbundle By Name(w1836) -> ("HBIN"=w1832:u16)
          n713 = Equal?(x=w1832, y=w1833) -> (x = y?=w1834:bool)
          n714 = case shown="True" w1834 {
            tunnel: [w1844 w1845] -> w1841
            tunnel: w1839 -> [w1844 w1846]
            frame False {
            }
            frame True {
              n715 = Increment(x=w1846) -> (x+1=w1845:i32)
            }
          }
        }
        frame 260 {
          n716 = Unbundle By Name(w1855) -> ("Interface.lvclass"=w1854:refnum<class "Interface.lvclass">)
          n717 = call "Read Camera Setup.vi"("Interface in"=w1854) -> ("Camera Setup"=w1848:T3)  [unwired: 8 in, 2 out]
          n718 = Unbundle By Name(w1848) -> ("VBIN"=w1847:u16)
          n719 = Number To Fractional String(number=w1847) -> (F-format string=w1849:string)  [unwired: 3 in]
          n720 = Concatenate Strings("SET VBIN " ("cmd"), w1849) -> (w1853:string)
          n721 = call-dynamic "Write cmd.vi"("error in (no error)"=w1857, "cmd"=w1853, "Device in"=w1855) -> ("error out"=w1856:errorcluster, "Device out"=w1858:refnum<class "Channel.lvclass">)  [unwired: 7 in]
          n722 = Increment(x=w1851) -> (x+1=w1852:i32)
        }
        frame 261 {
          n723 = call-dynamic "Read resp.vi"("error in (no error)"=w1866, "Device in"=w1867) -> ("error out"=w1860:errorcluster, "resp"=w1865:string, "Device out"=w1861:refnum<class "Channel.lvclass">)  [unwired: 7 in]
          n724 = Equal?(x=w1865, y="DONE") -> (x = y?=w1863:bool)
          n725 = case shown="True" w1863 {
            tunnel: [w1868 w1869] -> w1862
            tunnel: w1859 -> [w1868 w1870]
            frame False {
            }
            frame True {
              n726 = Increment(x=w1870) -> (x+1=w1869:i32)
            }
          }
        }
        frame 262 {
          n727 = call-dynamic "Write cmd.vi"("error in (no error)"=w1876, "cmd"="GET VBIN", "Device in"=w1874) -> ("error out"=w1875:errorcluster, "Device out"=w1877:refnum<class "Channel.lvclass">)  [unwired: 7 in]
          n728 = Increment(x=w1872) -> (x+1=w1873:i32)
        }
        frame 263 {
          n729 = call-dynamic "Read resp.vi"("error in (no error)"=w1888, "Device in"=w1889) -> ("error out"=w1886:errorcluster, "resp"=w1881:string, "Device out"=w1884:refnum<class "Channel.lvclass">)  [unwired: 7 in]
          n730 = Fract/Exp String To Number(string=w1881) -> (number=w1879:dbl)  [unwired: 3 in, 1 out]
          n731 = Unbundle By Name(w1884) -> ("Interface.lvclass"=w1883:refnum<class "Interface.lvclass">)
          n732 = call "Read Camera Setup.vi"("Interface in"=w1883) -> ("Camera Setup"=w1882:T3)  [unwired: 8 in, 2 out]
          n733 = Unbundle By Name(w1882) -> ("VBIN"=w1878:u16)
          n734 = Equal?(x=w1878, y=w1879) -> (x = y?=w1880:bool)
          n735 = case shown="True" w1880 {
            tunnel: [w1890 w1891] -> w1887
            tunnel: w1885 -> [w1890 w1892]
            frame False {
            }
            frame True {
              n736 = Increment(x=w1892) -> (x+1=w1891:i32)
            }
          }
        }
        frame 264 {
          n737 = Unbundle By Name(w1901) -> ("Interface.lvclass"=w1900:refnum<class "Interface.lvclass">)
          n738 = call "Read Camera Setup.vi"("Interface in"=w1900) -> ("Camera Setup"=w1894:T3)  [unwired: 8 in, 2 out]
          n739 = Unbundle By Name(w1894) -> ("INITIAL_LINE"=w1893:u16)
          n740 = Number To Fractional String(number=w1893) -> (F-format string=w1895:string)  [unwired: 3 in]
          n741 = Concatenate Strings("SET INITIAL_LINE " ("cmd"), w1895) -> (w1899:string)
          n742 = call-dynamic "Write cmd.vi"("error in (no error)"=w1903, "cmd"=w1899, "Device in"=w1901) -> ("error out"=w1902:errorcluster, "Device out"=w1904:refnum<class "Channel.lvclass">)  [unwired: 7 in]
          n743 = Increment(x=w1897) -> (x+1=w1898:i32)
        }
        frame 265 {
          n744 = call-dynamic "Read resp.vi"("error in (no error)"=w1912, "Device in"=w1913) -> ("error out"=w1906:errorcluster, "resp"=w1911:string, "Device out"=w1907:refnum<class "Channel.lvclass">)  [unwired: 7 in]
          n745 = Equal?(x=w1911, y="DONE") -> (x = y?=w1909:bool)
          n746 = case shown="True" w1909 {
            tunnel: [w1914 w1915] -> w1908
            tunnel: w1905 -> [w1914 w1916]
            frame False {
            }
            frame True {
              n747 = Increment(x=w1916) -> (x+1=w1915:i32)
            }
          }
        }
        frame 266 {
          n748 = call-dynamic "Write cmd.vi"("error in (no error)"=w1922, "cmd"="GET INITIAL_LINE", "Device in"=w1920) -> ("error out"=w1921:errorcluster, "Device out"=w1923:refnum<class "Channel.lvclass">)  [unwired: 7 in]
          n749 = Increment(x=w1918) -> (x+1=w1919:i32)
        }
        frame 267 {
          n750 = call-dynamic "Read resp.vi"("error in (no error)"=w1934, "Device in"=w1935) -> ("error out"=w1932:errorcluster, "resp"=w1927:string, "Device out"=w1930:refnum<class "Channel.lvclass">)  [unwired: 7 in]
          n751 = Fract/Exp String To Number(string=w1927) -> (number=w1925:dbl)  [unwired: 3 in, 1 out]
          n752 = Unbundle By Name(w1930) -> ("Interface.lvclass"=w1929:refnum<class "Interface.lvclass">)
          n753 = call "Read Camera Setup.vi"("Interface in"=w1929) -> ("Camera Setup"=w1928:T3)  [unwired: 8 in, 2 out]
          n754 = Unbundle By Name(w1928) -> ("INITIAL_LINE"=w1924:u16)
          n755 = Equal?(x=w1924, y=w1925) -> (x = y?=w1926:bool)
          n756 = case shown="True" w1926 {
            tunnel: [w1936 w1937] -> w1933
            tunnel: w1931 -> [w1936 w1938]
            frame False {
            }
            frame True {
              n757 = Increment(x=w1938) -> (x+1=w1937:i32)
            }
          }
        }
        frame 268 {
          n758 = Unbundle By Name(w1947) -> ("Interface.lvclass"=w1946:refnum<class "Interface.lvclass">)
          n759 = call "Read Camera Setup.vi"("Interface in"=w1946) -> ("Camera Setup"=w1940:T3)  [unwired: 8 in, 2 out]
          n760 = Unbundle By Name(w1940) -> ("INITIAL_COLUMN"=w1939:u16)
          n761 = Number To Fractional String(number=w1939) -> (F-format string=w1941:string)  [unwired: 3 in]
          n762 = Concatenate Strings("SET INITIAL_COLUMN " ("cmd"), w1941) -> (w1945:string)
          n763 = call-dynamic "Write cmd.vi"("error in (no error)"=w1949, "cmd"=w1945, "Device in"=w1947) -> ("error out"=w1948:errorcluster, "Device out"=w1950:refnum<class "Channel.lvclass">)  [unwired: 7 in]
          n764 = Increment(x=w1943) -> (x+1=w1944:i32)
        }
        frame 269 {
          n765 = call-dynamic "Read resp.vi"("error in (no error)"=w1958, "Device in"=w1959) -> ("error out"=w1952:errorcluster, "resp"=w1957:string, "Device out"=w1953:refnum<class "Channel.lvclass">)  [unwired: 7 in]
          n766 = Equal?(x=w1957, y="DONE") -> (x = y?=w1955:bool)
          n767 = case shown="True" w1955 {
            tunnel: [w1960 w1961] -> w1954
            tunnel: w1951 -> [w1960 w1962]
            frame False {
            }
            frame True {
              n768 = Increment(x=w1962) -> (x+1=w1961:i32)
            }
          }
        }
        frame 270 {
          n769 = call-dynamic "Write cmd.vi"("error in (no error)"=w1968, "cmd"="GET INITIAL_COLUMN", "Device in"=w1966) -> ("error out"=w1967:errorcluster, "Device out"=w1969:refnum<class "Channel.lvclass">)  [unwired: 7 in]
          n770 = Increment(x=w1964) -> (x+1=w1965:i32)
        }
        frame 271 {
          n771 = call-dynamic "Read resp.vi"("error in (no error)"=w1980, "Device in"=w1981) -> ("error out"=w1978:errorcluster, "resp"=w1973:string, "Device out"=w1976:refnum<class "Channel.lvclass">)  [unwired: 7 in]
          n772 = Fract/Exp String To Number(string=w1973) -> (number=w1971:dbl)  [unwired: 3 in, 1 out]
          n773 = Unbundle By Name(w1976) -> ("Interface.lvclass"=w1975:refnum<class "Interface.lvclass">)
          n774 = call "Read Camera Setup.vi"("Interface in"=w1975) -> ("Camera Setup"=w1974:T3)  [unwired: 8 in, 2 out]
          n775 = Unbundle By Name(w1974) -> ("INITIAL_COLUMN"=w1970:u16)
          n776 = Equal?(x=w1970, y=w1971) -> (x = y?=w1972:bool)
          n777 = case shown="True" w1972 {
            tunnel: [w1982 w1983] -> w1979
            tunnel: w1977 -> [w1982 w1984]
            frame False {
            }
            frame True {
              n778 = Increment(x=w1984) -> (x+1=w1983:i32)
            }
          }
        }
        frame 272 {
          n779 = Unbundle By Name(w1993) -> ("Interface.lvclass"=w1992:refnum<class "Interface.lvclass">)
          n780 = call "Read Camera Setup.vi"("Interface in"=w1992) -> ("Camera Setup"=w1986:T3)  [unwired: 8 in, 2 out]
          n781 = Unbundle By Name(w1986) -> ("FINAL_LINE"=w1985:u16)
          n782 = Number To Fractional String(number=w1985) -> (F-format string=w1987:string)  [unwired: 3 in]
          n783 = Concatenate Strings("SET FINAL_LINE " ("cmd"), w1987) -> (w1991:string)
          n784 = call-dynamic "Write cmd.vi"("error in (no error)"=w1995, "cmd"=w1991, "Device in"=w1993) -> ("error out"=w1994:errorcluster, "Device out"=w1996:refnum<class "Channel.lvclass">)  [unwired: 7 in]
          n785 = Increment(x=w1989) -> (x+1=w1990:i32)
        }
        frame 273 {
          n786 = call-dynamic "Read resp.vi"("error in (no error)"=w2004, "Device in"=w2005) -> ("error out"=w1998:errorcluster, "resp"=w2003:string, "Device out"=w1999:refnum<class "Channel.lvclass">)  [unwired: 7 in]
          n787 = Equal?(x=w2003, y="DONE") -> (x = y?=w2001:bool)
          n788 = case shown="True" w2001 {
            tunnel: [w2006 w2007] -> w2000
            tunnel: w1997 -> [w2006 w2008]
            frame False {
            }
            frame True {
              n789 = Increment(x=w2008) -> (x+1=w2007:i32)
            }
          }
        }
        frame 274 {
          n790 = call-dynamic "Write cmd.vi"("error in (no error)"=w2014, "cmd"="GET FINAL_LINE", "Device in"=w2012) -> ("error out"=w2013:errorcluster, "Device out"=w2015:refnum<class "Channel.lvclass">)  [unwired: 7 in]
          n791 = Increment(x=w2010) -> (x+1=w2011:i32)
        }
        frame 275 {
          n792 = call-dynamic "Read resp.vi"("error in (no error)"=w2026, "Device in"=w2027) -> ("error out"=w2024:errorcluster, "resp"=w2019:string, "Device out"=w2022:refnum<class "Channel.lvclass">)  [unwired: 7 in]
          n793 = Fract/Exp String To Number(string=w2019) -> (number=w2017:dbl)  [unwired: 3 in, 1 out]
          n794 = Unbundle By Name(w2022) -> ("Interface.lvclass"=w2021:refnum<class "Interface.lvclass">)
          n795 = call "Read Camera Setup.vi"("Interface in"=w2021) -> ("Camera Setup"=w2020:T3)  [unwired: 8 in, 2 out]
          n796 = Unbundle By Name(w2020) -> ("FINAL_LINE"=w2016:u16)
          n797 = Equal?(x=w2016, y=w2017) -> (x = y?=w2018:bool)
          n798 = case shown="True" w2018 {
            tunnel: [w2028 w2029] -> w2025
            tunnel: w2023 -> [w2028 w2030]
            frame False {
            }
            frame True {
              n799 = Increment(x=w2030) -> (x+1=w2029:i32)
            }
          }
        }
        frame 276 {
          n800 = Unbundle By Name(w2039) -> ("Interface.lvclass"=w2038:refnum<class "Interface.lvclass">)
          n801 = call "Read Camera Setup.vi"("Interface in"=w2038) -> ("Camera Setup"=w2032:T3)  [unwired: 8 in, 2 out]
          n802 = Unbundle By Name(w2032) -> ("FINAL_COLUMN"=w2031:u16)
          n803 = Number To Fractional String(number=w2031) -> (F-format string=w2033:string)  [unwired: 3 in]
          n804 = Concatenate Strings("SET FINAL_COLUMN " ("cmd"), w2033) -> (w2037:string)
          n805 = call-dynamic "Write cmd.vi"("error in (no error)"=w2041, "cmd"=w2037, "Device in"=w2039) -> ("error out"=w2040:errorcluster, "Device out"=w2042:refnum<class "Channel.lvclass">)  [unwired: 7 in]
          n806 = Increment(x=w2035) -> (x+1=w2036:i32)
        }
        frame 277 {
          n807 = call-dynamic "Read resp.vi"("error in (no error)"=w2050, "Device in"=w2051) -> ("error out"=w2044:errorcluster, "resp"=w2049:string, "Device out"=w2045:refnum<class "Channel.lvclass">)  [unwired: 7 in]
          n808 = Equal?(x=w2049, y="DONE") -> (x = y?=w2047:bool)
          n809 = case shown="True" w2047 {
            tunnel: [w2052 w2053] -> w2046
            tunnel: w2043 -> [w2052 w2054]
            frame False {
            }
            frame True {
              n810 = Increment(x=w2054) -> (x+1=w2053:i32)
            }
          }
        }
        frame 278 {
          n811 = call-dynamic "Write cmd.vi"("error in (no error)"=w2060, "cmd"="GET FINAL_COLUMN", "Device in"=w2058) -> ("error out"=w2059:errorcluster, "Device out"=w2061:refnum<class "Channel.lvclass">)  [unwired: 7 in]
          n812 = Increment(x=w2056) -> (x+1=w2057:i32)
        }
        frame 279 {
          n813 = call-dynamic "Read resp.vi"("error in (no error)"=w2072, "Device in"=w2073) -> ("error out"=w2070:errorcluster, "resp"=w2065:string, "Device out"=w2068:refnum<class "Channel.lvclass">)  [unwired: 7 in]
          n814 = Fract/Exp String To Number(string=w2065) -> (number=w2063:dbl)  [unwired: 3 in, 1 out]
          n815 = Unbundle By Name(w2068) -> ("Interface.lvclass"=w2067:refnum<class "Interface.lvclass">)
          n816 = call "Read Camera Setup.vi"("Interface in"=w2067) -> ("Camera Setup"=w2066:T3)  [unwired: 8 in, 2 out]
          n817 = Unbundle By Name(w2066) -> ("FINAL_COLUMN"=w2062:u16)
          n818 = Equal?(x=w2062, y=w2063) -> (x = y?=w2064:bool)
          n819 = disable-structure shown="Enabled" {
            disable-tunnel: [w2076 0 ("State")] -> w2071
            disable-tunnel: w2069 -> [w2075 _]
            disable-tunnel: w2064 -> [w2074 _]
            frame Disabled {
              n820 = case shown="True" w2074 {
                tunnel: [w2077 w2078] -> w2076
                tunnel: w2075 -> [w2077 w2079]
                frame False {
                }
                frame True {
                  n821 = Increment(x=w2079) -> (x+1=w2078:i32)
                }
              }
            }
            frame Enabled {
            }
          }
        }
        frame 280 {
          n822 = Unbundle By Name(w2089) -> ("Interface.lvclass"=w2088:refnum<class "Interface.lvclass">)
          n823 = call "Read Camera Setup.vi"("Interface in"=w2088) -> ("Camera Setup"=w2082:T3)  [unwired: 8 in, 2 out]
          n824 = Unbundle By Name(w2082) -> ("VERTICAL_CLOCK_VOLTAGE"=w2081:u8)
          n825 = Number To Fractional String(number=w2081) -> (F-format string=w2083:string)  [unwired: 3 in]
          n826 = Concatenate Strings("SET VERTICAL_CLOCK_VOLTAGE " ("cmd"), w2083) -> (w2087:string)
          n827 = call-dynamic "Write cmd.vi"("error in (no error)"=w2091, "cmd"=w2087, "Device in"=w2089) -> ("error out"=w2090:errorcluster, "Device out"=w2092:refnum<class "Channel.lvclass">)  [unwired: 7 in]
          n828 = Increment(x=w2085) -> (x+1=w2086:i32)
        }
        frame 281 {
          n829 = call-dynamic "Read resp.vi"("error in (no error)"=w2100, "Device in"=w2101) -> ("error out"=w2094:errorcluster, "resp"=w2099:string, "Device out"=w2095:refnum<class "Channel.lvclass">)  [unwired: 7 in]
          n830 = Equal?(x=w2099, y="DONE") -> (x = y?=w2097:bool)
          n831 = case shown="True" w2097 {
            tunnel: [w2102 w2103] -> w2096
            tunnel: w2093 -> [w2102 w2104]
            frame False {
            }
            frame True {
              n832 = Increment(x=w2104) -> (x+1=w2103:i32)
            }
          }
        }
        frame 282 {
          n833 = call-dynamic "Write cmd.vi"("error in (no error)"=w2110, "cmd"="GET VERTICAL_CLOCK_VOLTAGE", "Device in"=w2108) -> ("error out"=w2109:errorcluster, "Device out"=w2111:refnum<class "Channel.lvclass">)  [unwired: 7 in]
          n834 = Increment(x=w2106) -> (x+1=w2107:i32)
        }
        frame 283 {
          n835 = call-dynamic "Read resp.vi"("error in (no error)"=w2122, "Device in"=w2123) -> ("error out"=w2120:errorcluster, "resp"=w2115:string, "Device out"=w2118:refnum<class "Channel.lvclass">)  [unwired: 7 in]
          n836 = Fract/Exp String To Number(string=w2115) -> (number=w2113:dbl)  [unwired: 3 in, 1 out]
          n837 = Unbundle By Name(w2118) -> ("Interface.lvclass"=w2117:refnum<class "Interface.lvclass">)
          n838 = call "Read Camera Setup.vi"("Interface in"=w2117) -> ("Camera Setup"=w2116:T3)  [unwired: 8 in, 2 out]
          n839 = Unbundle By Name(w2116) -> ("VERTICAL_CLOCK_VOLTAGE"=w2112:u8)
          n840 = Equal?(x=w2112, y=w2113) -> (x = y?=w2114:bool)
          n841 = case shown="True" w2114 {
            tunnel: [w2124 w2125] -> w2121
            tunnel: w2119 -> [w2124 w2126]
            frame False {
            }
            frame True {
              n842 = Increment(x=w2126) -> (x+1=w2125:i32)
            }
          }
        }
        frame 284 {
          n843 = Unbundle By Name(w2135) -> ("Interface.lvclass"=w2134:refnum<class "Interface.lvclass">)
          n844 = call "Read Camera Setup.vi"("Interface in"=w2134) -> ("Camera Setup"=w2129:T3)  [unwired: 8 in, 2 out]
          n845 = Unbundle By Name(w2129) -> ("FRAME_TRANSFER"=w2128:bool)
          n846 = case shown="True" w2128 {
            tunnel: ["T" ("cmd") "F" ("cmd")] -> w2127
            frame True {
            }
            frame False {
            }
          }
          n847 = Concatenate Strings("SET FRAME_TRANSFER " ("cmd"), w2127) -> (w2133:string)
          n848 = call-dynamic "Write cmd.vi"("error in (no error)"=w2137, "cmd"=w2133, "Device in"=w2135) -> ("error out"=w2136:errorcluster, "Device out"=w2138:refnum<class "Channel.lvclass">)  [unwired: 7 in]
          n849 = Increment(x=w2131) -> (x+1=w2132:i32)
        }
        frame 285 {
          n850 = call-dynamic "Read resp.vi"("error in (no error)"=w2148, "Device in"=w2149) -> ("error out"=w2142:errorcluster, "resp"=w2147:string, "Device out"=w2143:refnum<class "Channel.lvclass">)  [unwired: 7 in]
          n851 = Equal?(x=w2147, y="DONE") -> (x = y?=w2145:bool)
          n852 = case shown="True" w2145 {
            tunnel: [w2150 w2151] -> w2144
            tunnel: w2141 -> [w2150 w2152]
            frame False {
            }
            frame True {
              n853 = Increment(x=w2152) -> (x+1=w2151:i32)
            }
          }
        }
        frame 286 {
          n854 = call-dynamic "Write cmd.vi"("error in (no error)"=w2158, "cmd"="GET FRAME_TRANSFER", "Device in"=w2156) -> ("error out"=w2157:errorcluster, "Device out"=w2159:refnum<class "Channel.lvclass">)  [unwired: 7 in]
          n855 = Increment(x=w2154) -> (x+1=w2155:i32)
        }
        frame 287 {
          n856 = call-dynamic "Read resp.vi"("error in (no error)"=w2170, "Device in"=w2171) -> ("error out"=w2168:errorcluster, "resp"=w2162:string, "Device out"=w2166:refnum<class "Channel.lvclass">)  [unwired: 7 in]
          n857 = Unbundle By Name(w2166) -> ("Interface.lvclass"=w2165:refnum<class "Interface.lvclass">)
          n858 = call "Read Camera Setup.vi"("Interface in"=w2165) -> ("Camera Setup"=w2164:T3)  [unwired: 8 in, 2 out]
          n859 = Unbundle By Name(w2164) -> ("FRAME_TRANSFER"=w2161:bool)
          n860 = case shown="True" w2161 {
            tunnel: ["T" "F"] -> w2160
            frame True {
            }
            frame False {
            }
          }
          n861 = Equal?(x=w2160, y=w2162) -> (x = y?=w2163:bool)
          n862 = case shown="True" w2163 {
            tunnel: [w2174 w2175] -> w2169
            tunnel: w2167 -> [w2174 w2176]
            frame False {
            }
            frame True {
              n863 = Increment(x=w2176) -> (x+1=w2175:i32)
            }
          }
        }
        frame 288 {
          n864 = Unbundle By Name(w2185) -> ("Interface.lvclass"=w2184:refnum<class "Interface.lvclass">)
          n865 = call "Read Camera Setup.vi"("Interface in"=w2184) -> ("Camera Setup"=w2178:T3)  [unwired: 8 in, 2 out]
          n866 = Unbundle By Name(w2178) -> ("AD_CHANNEL"=w2177:u32)
          n867 = Number To Fractional String(number=w2177) -> (F-format string=w2179:string)  [unwired: 3 in]
          n868 = Concatenate Strings("SET AD_CHANNEL " ("cmd"), w2179) -> (w2183:string)
          n869 = call-dynamic "Write cmd.vi"("error in (no error)"=w2187, "cmd"=w2183, "Device in"=w2185) -> ("error out"=w2186:errorcluster, "Device out"=w2188:refnum<class "Channel.lvclass">)  [unwired: 7 in]
          n870 = Increment(x=w2181) -> (x+1=w2182:i32)
        }
        frame 289 {
          n871 = call-dynamic "Read resp.vi"("error in (no error)"=w2196, "Device in"=w2197) -> ("error out"=w2190:errorcluster, "resp"=w2195:string, "Device out"=w2191:refnum<class "Channel.lvclass">)  [unwired: 7 in]
          n872 = Equal?(x=w2195, y="DONE") -> (x = y?=w2193:bool)
          n873 = case shown="True" w2193 {
            tunnel: [w2198 w2199] -> w2192
            tunnel: w2189 -> [w2198 w2200]
            frame False {
            }
            frame True {
              n874 = Increment(x=w2200) -> (x+1=w2199:i32)
            }
          }
        }
        frame 290 {
          n875 = call-dynamic "Write cmd.vi"("error in (no error)"=w2206, "cmd"="GET AD_CHANNEL", "Device in"=w2204) -> ("error out"=w2205:errorcluster, "Device out"=w2207:refnum<class "Channel.lvclass">)  [unwired: 7 in]
          n876 = Increment(x=w2202) -> (x+1=w2203:i32)
        }
        frame 291 {
          n877 = call-dynamic "Read resp.vi"("error in (no error)"=w2218, "Device in"=w2219) -> ("error out"=w2216:errorcluster, "resp"=w2211:string, "Device out"=w2214:refnum<class "Channel.lvclass">)  [unwired: 7 in]
          n878 = Fract/Exp String To Number(string=w2211) -> (number=w2209:dbl)  [unwired: 3 in, 1 out]
          n879 = Unbundle By Name(w2214) -> ("Interface.lvclass"=w2213:refnum<class "Interface.lvclass">)
          n880 = call "Read Camera Setup.vi"("Interface in"=w2213) -> ("Camera Setup"=w2212:T3)  [unwired: 8 in, 2 out]
          n881 = Unbundle By Name(w2212) -> ("AD_CHANNEL"=w2208:u32)
          n882 = Equal?(x=w2208, y=w2209) -> (x = y?=w2210:bool)
          n883 = case shown="True" w2210 {
            tunnel: [w2220 w2221] -> w2217
            tunnel: w2215 -> [w2220 w2222]
            frame False {
            }
            frame True {
              n884 = Increment(x=w2222) -> (x+1=w2221:i32)
            }
          }
        }
      }
      n885 = call-dynamic "Read State Machine.vi"("error in (no error)"=w7, "Device in"=w14) -> ("error out"=w10:errorcluster, "State Machine.lvclass"=w13:refnum<class "State Machine.lvclass">, "Device out"=w12:refnum<class "Channel.lvclass">)  [unwired: 7 in]
      n886 = call "Next State.vi"("error in (no error)"=w10, "New_State"=w8, "State Machine in"=w13) -> ("error out"=w9:errorcluster, "State Machine out"=w15:refnum<class "State Machine.lvclass">)  [unwired: 7 in]
      n887 = call-dynamic "Write State Machine.vi"("error in (no error)"=w9, "State Machine.lvclass"=w15, "Device in"=w12) -> ("error out"=w6:errorcluster, "Device out"=w11:refnum<class "Channel.lvclass">)  [unwired: 7 in]
    }
    frame Error {
    }
  }
  "error out" <- w3
  "Channel out" <- w1
